vi "Run Test - Stop Condition (SubVI).vi"(8 "error in (no error)":errorcluster, 9 "Time":dbl, 11 "Cluster in":T2 {"M Event" items=["Stop", "Running", "PID", "Up Limit", "Down Limit", "Load Limit"]; "Test Type" items=["Please Select", "Triaxial Shear", "Triaxial UU", "Shearbox", "Permeability", "Consolidation (Stepped Loading)/Swelling", "Saturation (Incremental)", "User Defined", "UCT", "Isotropic Consolidation", "Swelling Pressure"]; "Data"."Test Type" items=["Please Select", "Triaxial Shear", "Triaxial UU", "Shearbox", "Permeability", "Consolidation (Stepped Loading)/Swelling", "Saturation (Incremental)", "User Defined", "UCT", "Isotropic Consolidation", "Swelling Pressure"]}) -> (0 "error out":errorcluster, 1 "Perm":T1, 2 "Delay":string, 3 "Cluster out":T2 {"M Event" items=["Stop", "Running", "PID", "Up Limit", "Down Limit", "Load Limit"]; "Test Type" items=["Please Select", "Triaxial Shear", "Triaxial UU", "Shearbox", "Permeability", "Consolidation (Stepped Loading)/Swelling", "Saturation (Incremental)", "User Defined", "UCT", "Isotropic Consolidation", "Swelling Pressure"]; "Data"."Test Type" items=["Please Select", "Triaxial Shear", "Triaxial UU", "Shearbox", "Permeability", "Consolidation (Stepped Loading)/Swelling", "Saturation (Incremental)", "User Defined", "UCT", "Isotropic Consolidation", "Swelling Pressure"]}, 5 "Enum":T11)   [LabVIEW 2019]
uses:
  Controls/RunTest - State.ctl
  Controls/RunTest - Data Structure.ctl
  Controls/Test Panel - Data Structure.ctl
  Controls/Station - Test Type.ctl
  <vilib>/Utility/miscctls.llb/LVRowAndColumnTypeDef.ctl
  Controls/RunTest - Calculate Data.ctl
  <vilib>/httpClient/ClientHandle.ctl
  Controls/RunTest - Start Condition.ctl
  Controls/RunTest - Stop Condition.ctl
  Controls/UDP - Event.ctl
  Controls/eFGV States.ctl
  <vilib>/httpClient/LabVIEWHTTPClient.lvlib
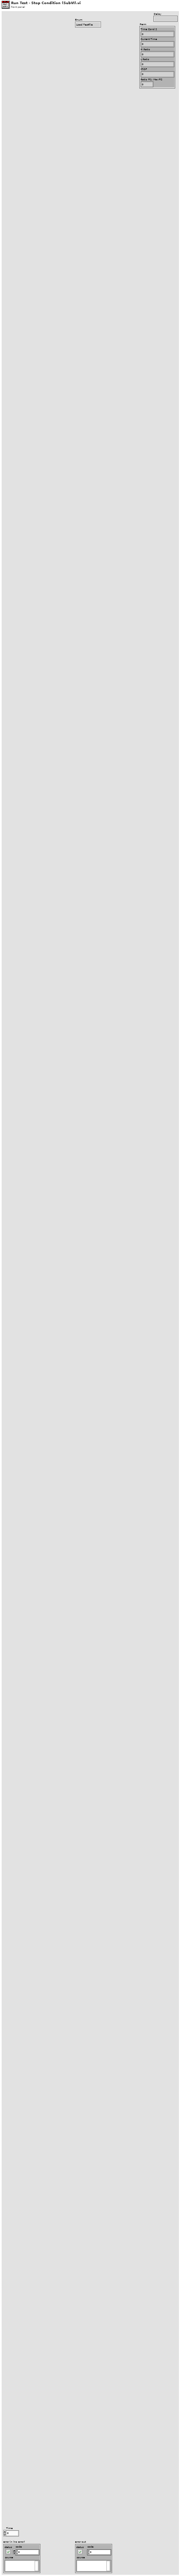
[diagram p1: front panel]
types:
  T1 = cluster{"Time Cond 2":dbl, "Current Time":dbl, "H Ratio":dbl, "L Ratio":dbl, "IF/OF":dbl, "Ratio =1; Max=2":u32}
  T2 = typedef "RunTest - Data Structure.ctl" = cluster{"Test Plan":string[], "PlanRow":i32, "Device Name":string[], "Timeout":i32, "Start?":bool, "Pause?":bool, "IP Address":string[], "LogRow":i32, "Logtype":u16, "Log Elapse":sgl, "Data":T3, "Stop log?":bool, "tdms":refnum<k34>, "Sensor Data":sgl[], "Start time":timestamp, "Prev Log Elapse":u32, "Plot":u16, "X-Axis":u16[], "Y-Axis":u16[], "XY":cluster{"X":dbl, "Y":dbl}[][], "End Stage?":bool, "1run":bool, "Condition":u16[], "Start Con":bool, "Log Con":bool, "Stop Con":bool, "Start Elapse":dbl, "Start Load":dbl, "Motor":i32, "StartRow":i32, "number log":i32, "Dir":bool, "Start time test":timestamp, "Auto":bool, "Check return?":bool, "Inv":cluster{"M":i32[], "Bool":bool[]}, "tdms temp":refnum<k34>, "Zero?":bool, "Plot Timer":dbl, "1st Run":bool, "TDMS Path":path, "MaxLoad":dbl, "Log Timer":sgl[], "Test Type":T4, "Log Sensor":string[], "Save?":bool, "1st Log":bool, "Y-Axis 2":u16[], "On Y-Axis 2":bool, "Decimal":u8[], "Init":cluster{"PWP TS":sgl, "Load TS":sgl, "Volume TS":sgl, "Disp TS":sgl, "CP":sgl, "Vol In":sgl, "Vol Out":sgl, "Load UCT":sgl, "Disp UCT":sgl, "PWP Sat":sgl, "CP Sat":sgl, "Volume IsoCons":sgl, "PWP IsoCons":sgl, "PWP TUU":sgl, "Load TUU":sgl, "Volume TUU":sgl, "Disp TUU":sgl, "Load Cons":sgl, "Disp Cons":sgl, "Volume Sat":sgl, "Vertical Load SB":sgl, "Vertical Disp SB":sgl, "H Disp SB":sgl, "H Load SB":sgl}, "Calc":T6, "Device Index":i32[], "Channel Index":i32[], "http ref":T7, "fileid":string, "Step Cons":cluster{"V Stress":sgl, "H Settlement":sgl}, "RunTest":bool, "Graph Last":i32, "Init?":bool, "Datalog":bool[], "Start":T8, "Stop":T9, "Running?":bool, "StartTime":dbl, "Log Prev Time":dbl, "KeyName":string[], "Test RunTime":dbl, "Log Prev Axial":dbl, "M Event":T10[], "Last Log":bool, "popup":bool, "PreStart UU":bool, "PreStart Sat":bool}
  T3 = typedef "Test Panel - Data Structure.ctl" = cluster{"Station":string, "Sample ID":string, "Job No":string, "Job Description":string, "Filename":string, "Test Type":T4, "Speciment No":string, "Depth":string, "Height":string, "Diameter/Length":string, "Weight":string, "Test Parameter":string, "Station[]":string[], "Edit Pos":T5, "Edit Pos Prev":T5, "Area":string, "Path":string}
  T4 = typedef "Station - Test Type.ctl" = u16
  T5 = typedef "LVRowAndColumnTypeDef.ctl" = cluster{"Row":i32, "Column":i32}
  T6 = typedef "RunTest - Calculate Data.ctl" = cluster{"TS":cluster{"Change PWP":sgl, "Change Vol":sgl, "Axial Load":sgl, "CiL":sgl, "Deviator":sgl, "Axial Strain":sgl, "MaxDeviator":sgl}, "TUU":cluster{"Change PWP":sgl, "Axial Load":sgl, "CiL":sgl, "Deviator":sgl, "Axial Strain":sgl, "MaxDeviator":sgl}, "Sat":cluster{"B Value":sgl, "PWP Diss":sgl, "CPP":sgl, "CV":sgl}, "Per":cluster{"Change Vol In":sgl, "Change Vol Out":sgl, "Mean Vol":sgl, "Gradient Pressure":sgl, "Outlet Flow":sgl, "Inlet Flow":sgl, "I X1":sgl, "I X2":sgl, "I Y1":sgl, "I Y2":sgl, "O X1":sgl, "O X2":sgl, "O Y1":sgl, "O Y2":sgl}, "Step Cons":cluster{"V Stress":sgl, "H Settlement":sgl, "Total H Settle":sgl, "Prev Total H":sgl}, "UCT":cluster{"ALC":sgl, "H Change":sgl, "Deviator":sgl, "Axial Strain":sgl, "V Stress":sgl, "MaxDeviator":sgl}, "ISO Cons":cluster{"CPP":sgl, "PWP Diss":sgl, "CV":sgl}, "SB":cluster{"Speci LenC":sgl, "Shear Strain":sgl, "H LC":sgl, "Normal Stress":sgl, "Shear Stress":sgl, "MaxShear":sgl}}
  T7 = typedef "LabVIEWHTTPClient.lvlib/ClientHandle.ctl" = refnum<k1>
  T8 = typedef "RunTest - Start Condition.ctl" = cluster{"Cons":cluster{"VS":dbl, "Delay":bool, "No Delay":dbl}, "Sat":cluster{"CP":dbl, "BP":dbl, "StartBP":bool, "Target CP":bool, "Target BP":bool}, "Iso":cluster{"Select":dbl, "BP":dbl, "IC2":dbl, "IC3":dbl, "IC4":dbl, ". IC6":bool, "IC6":dbl, "IC6-2":dbl, "Target":bool, "Time Cond":dbl, "Last PWP":dbl}, "TS":cluster{"SS":dbl, "Engage":bool, "ES":dbl, "LC":dbl, "PreStart":bool, "Trig SS":bool, "Drain":dbl}, "TUU":cluster{"SS":dbl, "Engage":bool, "ES":dbl, "LC":dbl, "PreStart":bool, "Trig SS":bool, "CP":dbl, "Delay Value":dbl, "Delay":bool, "CP PID":bool}, "UCT":cluster{"SS":dbl, "Engage":bool, "ES":dbl, "LC":dbl, "PreStart":bool, "Trig SS":bool}, "Enable?":bool, "SB":cluster{"SS":dbl, "Engage":bool, "ES":dbl, "LC":dbl, "PreStart":bool, "Trig SS":bool, "VS":dbl, "Delay Value":dbl, "Delay":bool, "VS PID":bool}, "Perm":cluster{"DP":dbl}}
  T9 = typedef "RunTest - Stop Condition.ctl" = cluster{"Cons":cluster{"Select":i32, "Disp":dbl, "Time":dbl, "Time2":dbl, "Disp 2":dbl, "Time Cond":dbl, "Last Disp":dbl, "Swell":bool}, "Sat":cluster{"Select":i32, "PP":dbl, "Time":dbl, "VC":dbl, "Time2":dbl, "Time Cond":dbl, "Last PP":dbl, ".B":bool, "B":dbl, "Last Vc":dbl, "Time Cond 2":dbl, "Time3":dbl, "Time Cond 3":dbl, "B Achieve":bool}, "Iso":cluster{"PP":dbl, "Time":dbl, "VC":dbl, "Time2":dbl, "Time Cond":dbl, "Last Vc":dbl, ".PP":bool, "Time Cond 2":dbl, "Select":i32}, "TS":cluster{"Axial":dbl, ".MaxDev":bool, "MaxDev Value":dbl, "Return":bool, "Reset":bool, "Prev Time":dbl, "PostStop Run":bool, "CP Stop":bool, "BP Stop":bool, "PostStop Trig":bool, "Reset Value":dbl, "BPTrig":bool, "CPTrig":bool, "VLCTrig":bool}, "TUU":cluster{"Axial":dbl, ".MaxDev":bool, "MaxDev Value":dbl, "Return":bool, "Reset":bool, "Prev Time":dbl, "PostStop Run":bool, "CP Stop":bool, "BP Stop":bool, "PostStop Trig":bool, "Reset Value":dbl, "BPTrig":bool, "CPTrig":bool, "VLCTrig":bool}, "UCT":cluster{"Axial":dbl, ".MaxDev":bool, "MaxDev Value":dbl, "Return":bool, "Reset":bool, "Prev Time":dbl, "PostStop Run":bool, "CP Stop":bool, "BP Stop":bool, "PostStop Trig":bool}, "Enable?":bool, "SB":cluster{"Shear":dbl, ".MaxShear":bool, "MaxShear Value":dbl, "Return":bool, "Reset":bool, "Prev Time":dbl, "PostStop Run":bool, "CP Stop":bool, "BP Stop":bool, "PostStop Trig":bool, "Reset Value":dbl, "BPTrig":bool, "CPTrig":bool, "VLCTrig":bool}, "Perm":cluster{"Max Time":bool, "Reset":bool, "PostStop Run":bool, "Ratio":bool, "Reset Value":dbl, "Time":dbl, "RatioTime":dbl, "RatioMore":dbl, "RatioLess":dbl, "Time Cond":dbl, "Time Cond 2":dbl, "Prev IF":dbl, "Prev OF":dbl, "PostStop Trig":bool, "BP Trig":bool, "DP Stop":bool, "BP Stop":bool, "CP Stop":bool, "CP Trig":bool}, "SP":cluster{".Max Time":bool, ".Time":bool, "Time":dbl, "MaxTime":dbl, "Time Cond":dbl, "Max Time Cond":dbl, "Stress":dbl}}
  T10 = typedef "UDP - Event.ctl" = u16
  T11 = typedef "RunTest - State.ctl" = enum16{"Load Testfile", "Notifier", "Init", "Idle", "Load", "Read DB", "Run", "Pause", "Stop", "Check Start", "Check Stop", "Check Post Stop", "Check Log", "EndStage", "Data View", "Display", "Graph", "Graph Old", "Close", "Stop PID", "Check Limit", "Auto", "Up", "Log", "Zero", "Machine Control", "Save Report"}
  T12 = typedef "eFGV States.ctl" = enum16{"Init", "Read", "Write", "Exit"}
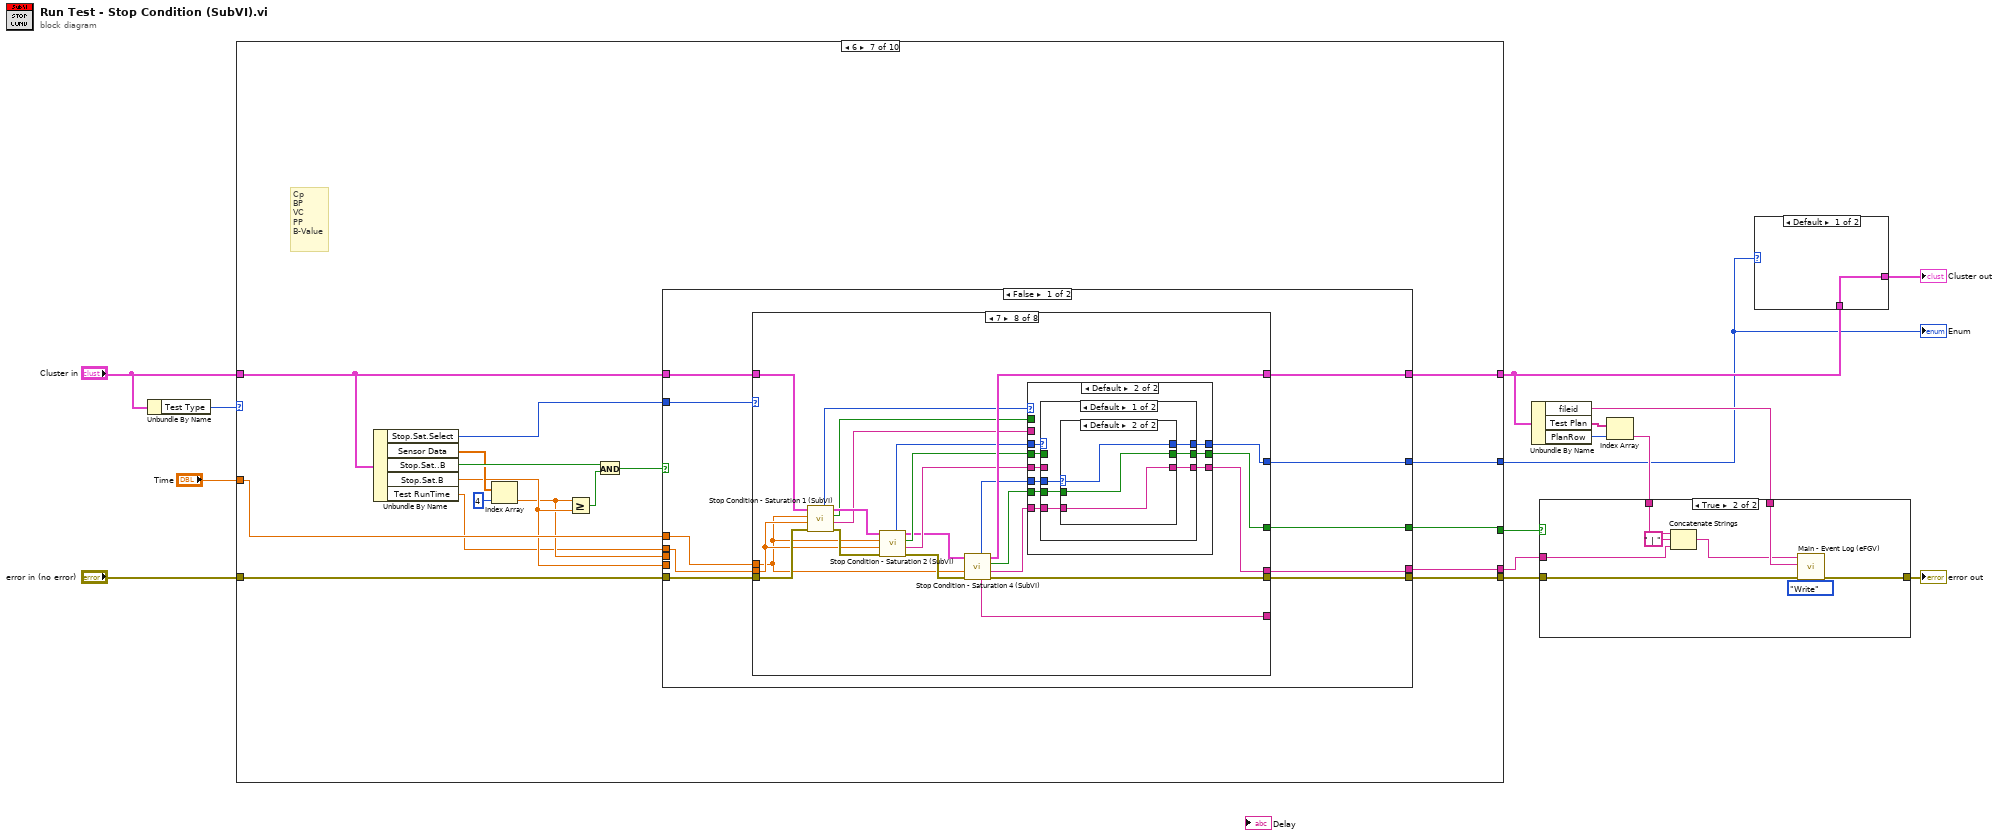
[diagram p0: block diagram]
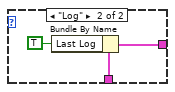
[diagram p2: hidden frame]
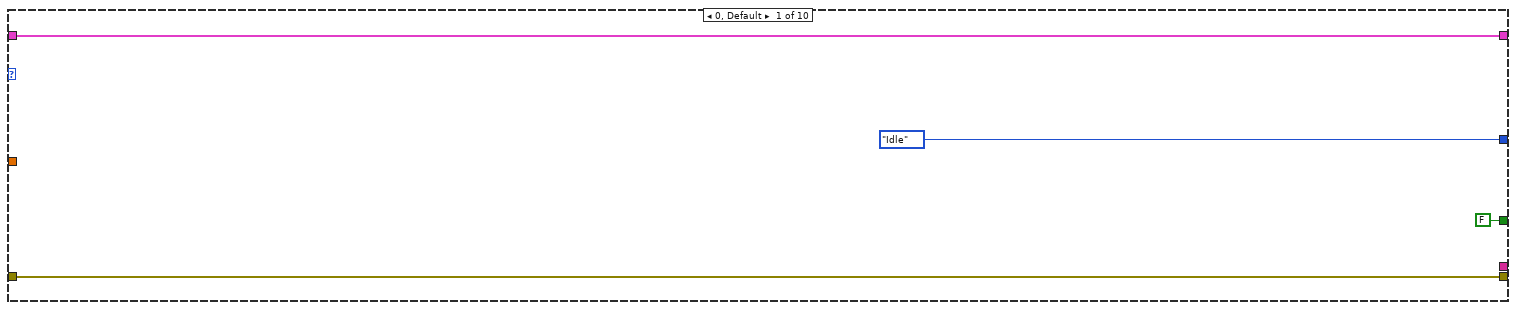
[diagram p3: hidden frame]
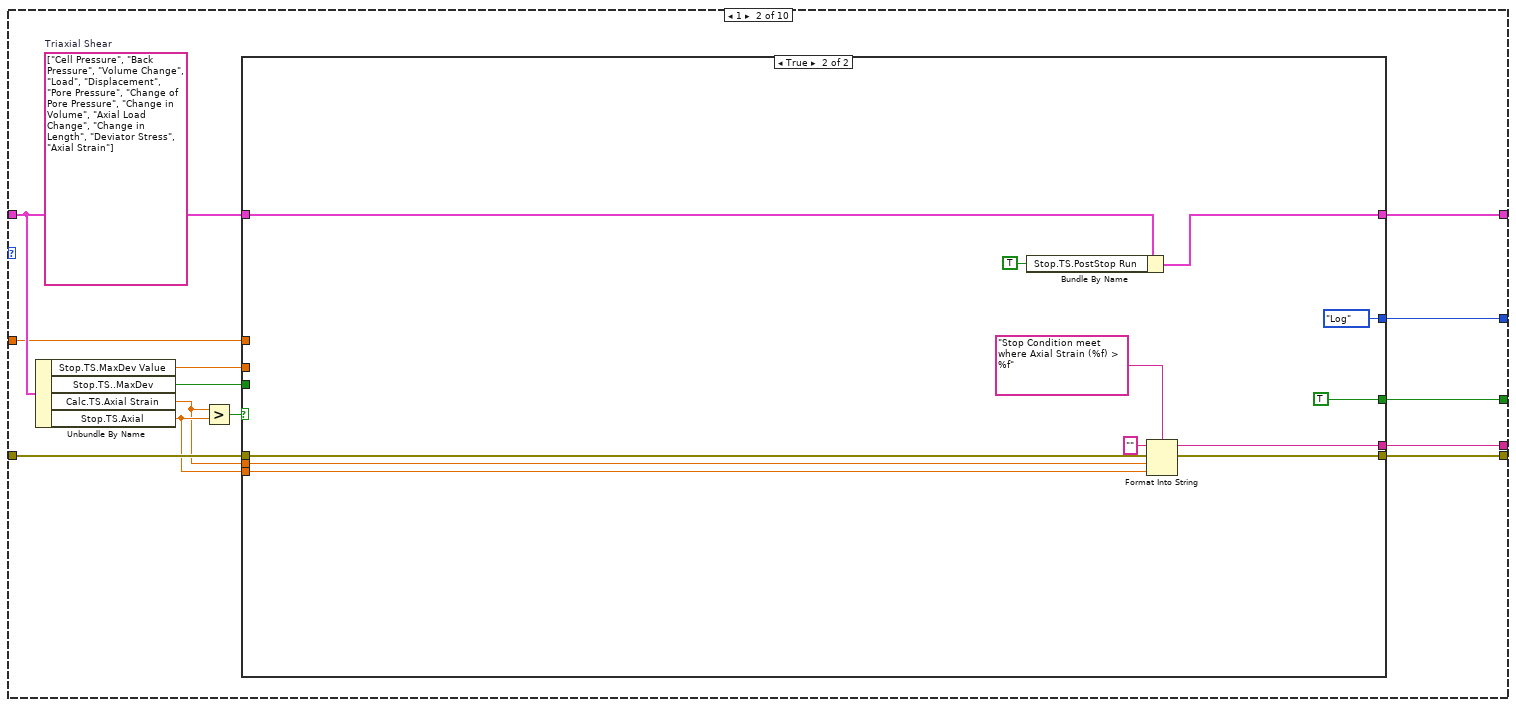
[diagram p4: hidden frame]
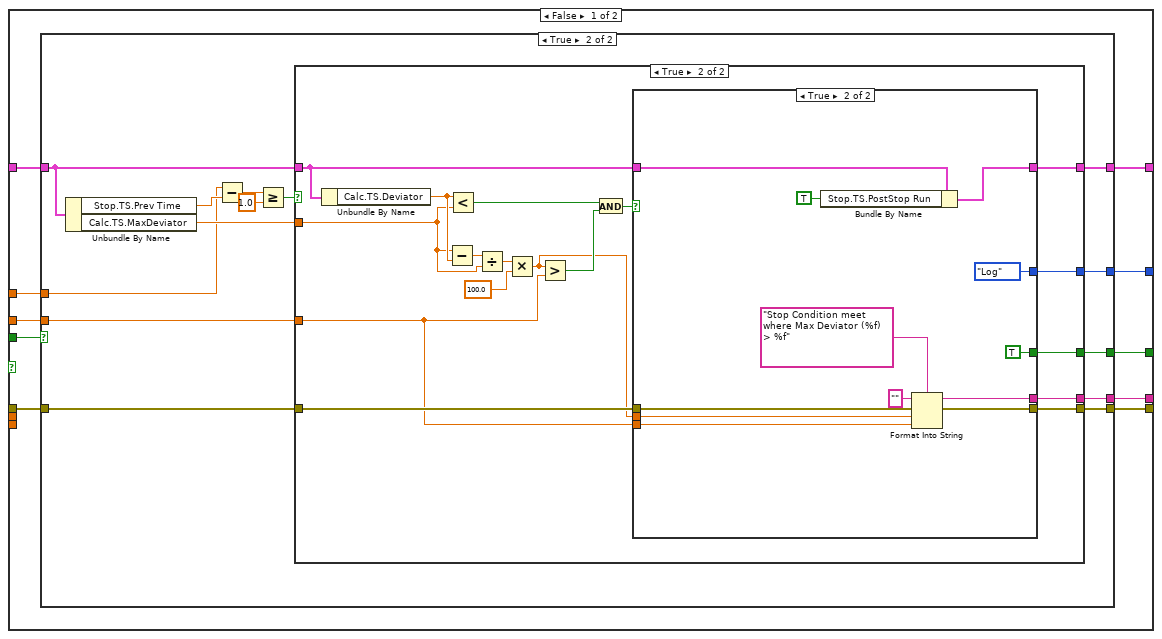
[diagram p5: hidden frame]
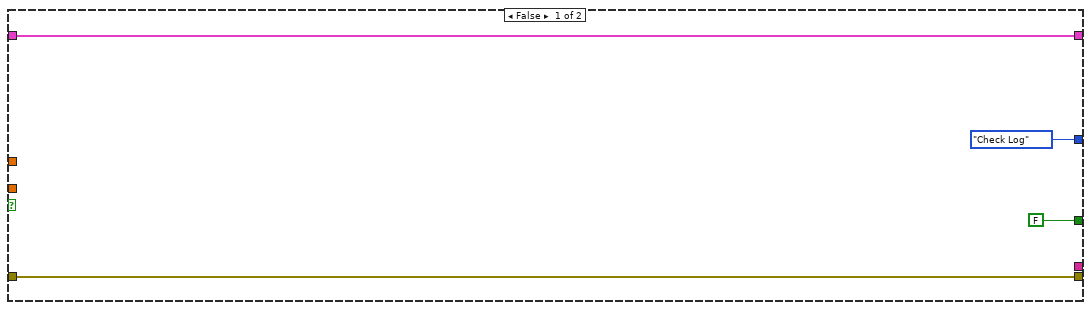
[diagram p6: hidden frame]
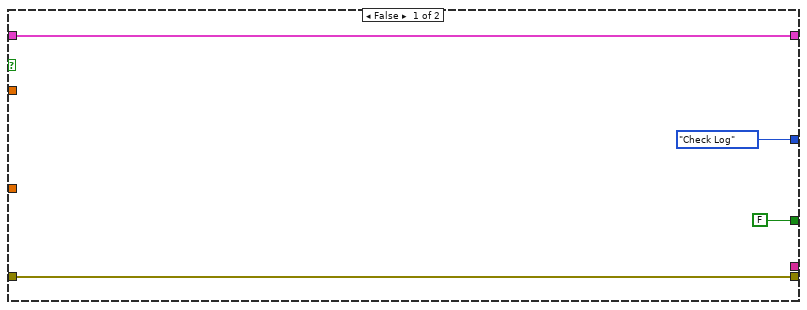
[diagram p7: hidden frame]
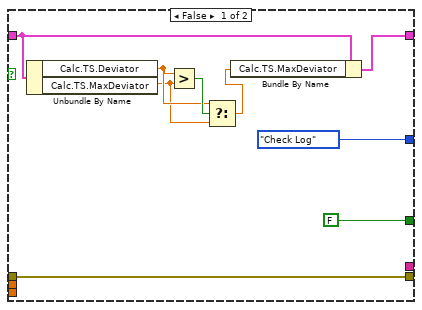
[diagram p8: hidden frame]
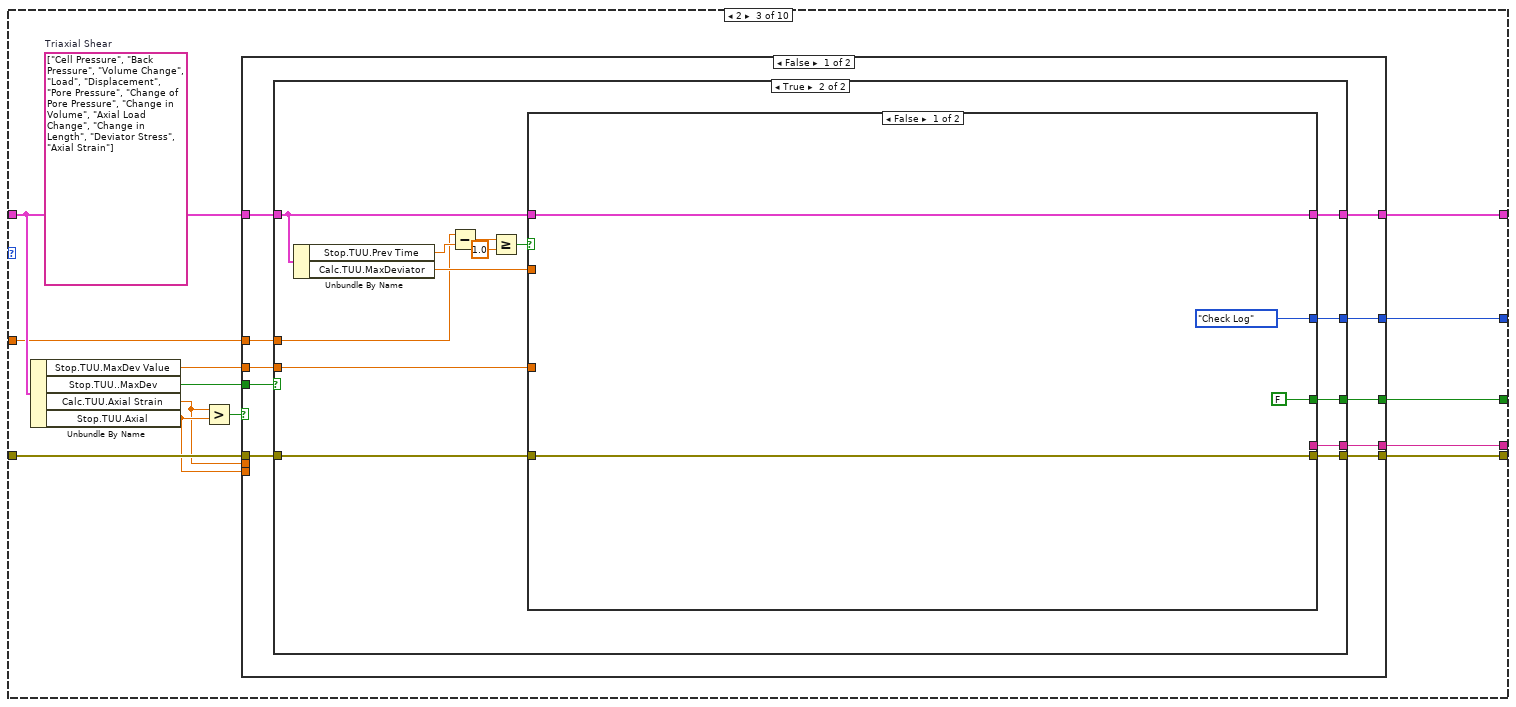
[diagram p9: hidden frame]
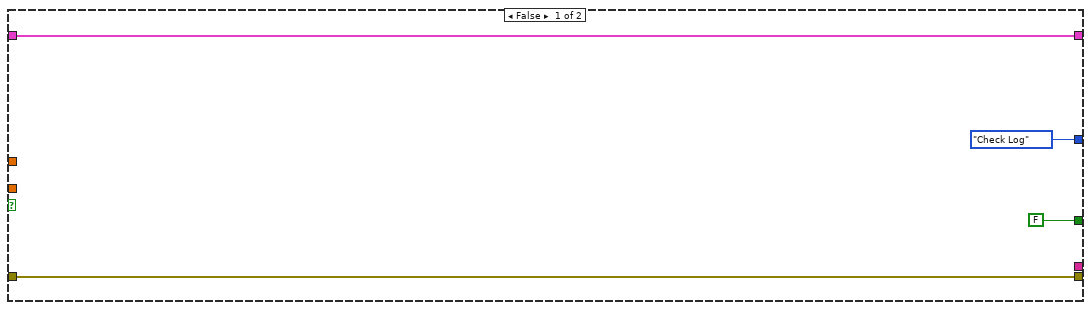
[diagram p10: hidden frame]
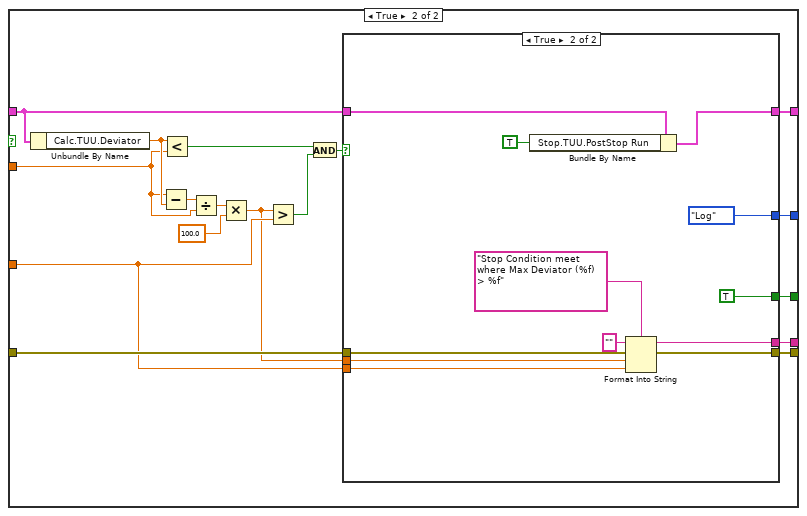
[diagram p11: hidden frame]
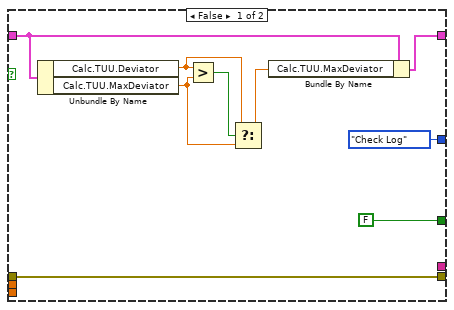
[diagram p12: hidden frame]
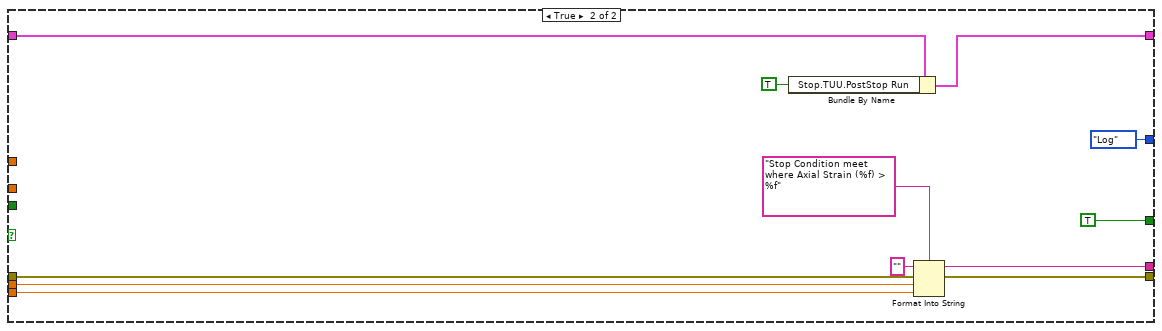
[diagram p13: hidden frame]
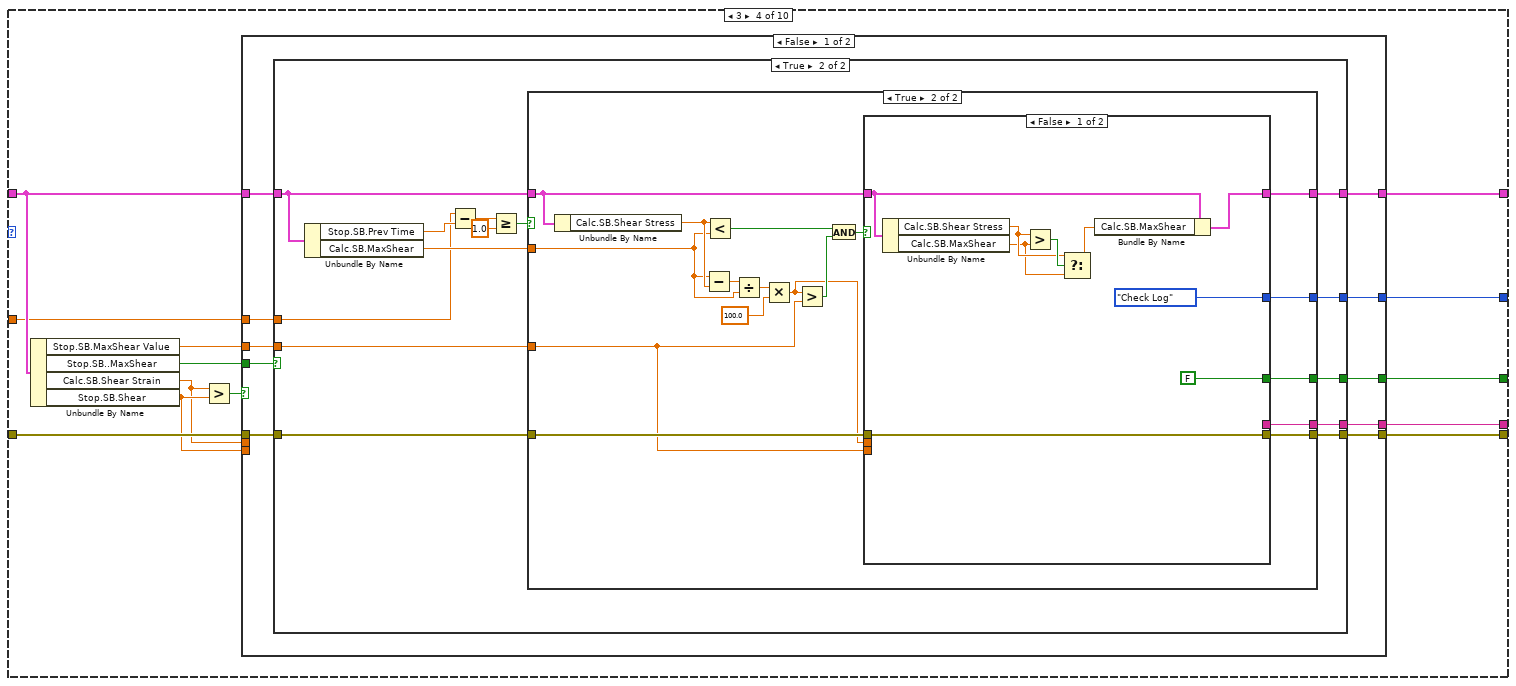
[diagram p14: hidden frame]
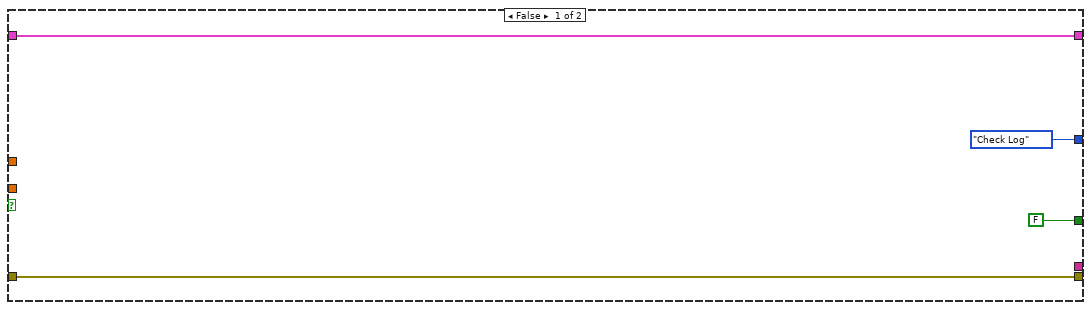
[diagram p15: hidden frame]
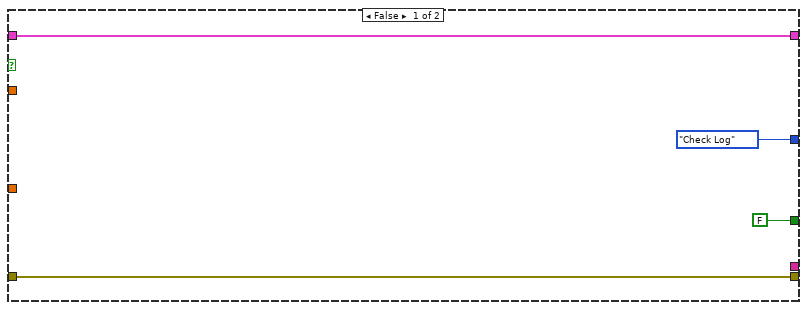
[diagram p16: hidden frame]
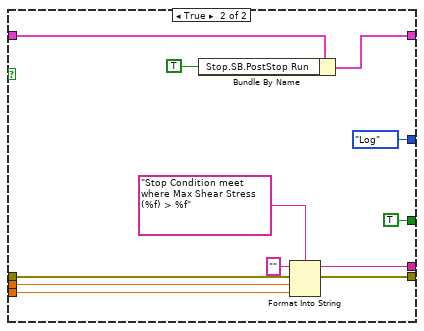
[diagram p17: hidden frame]
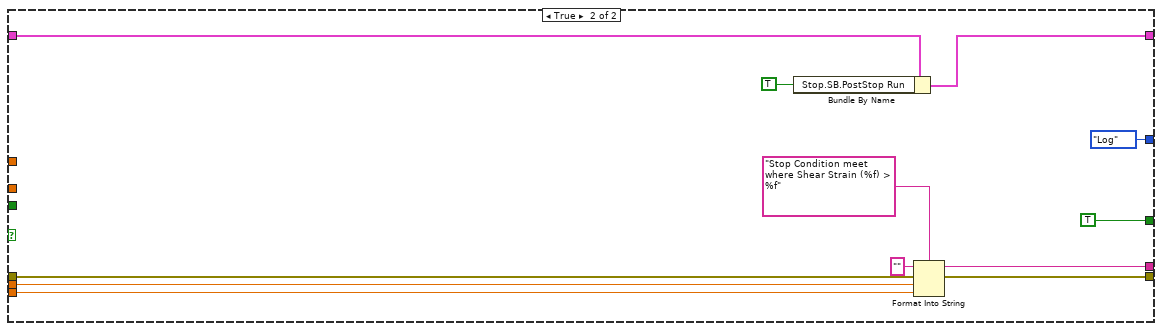
[diagram p18: hidden frame]
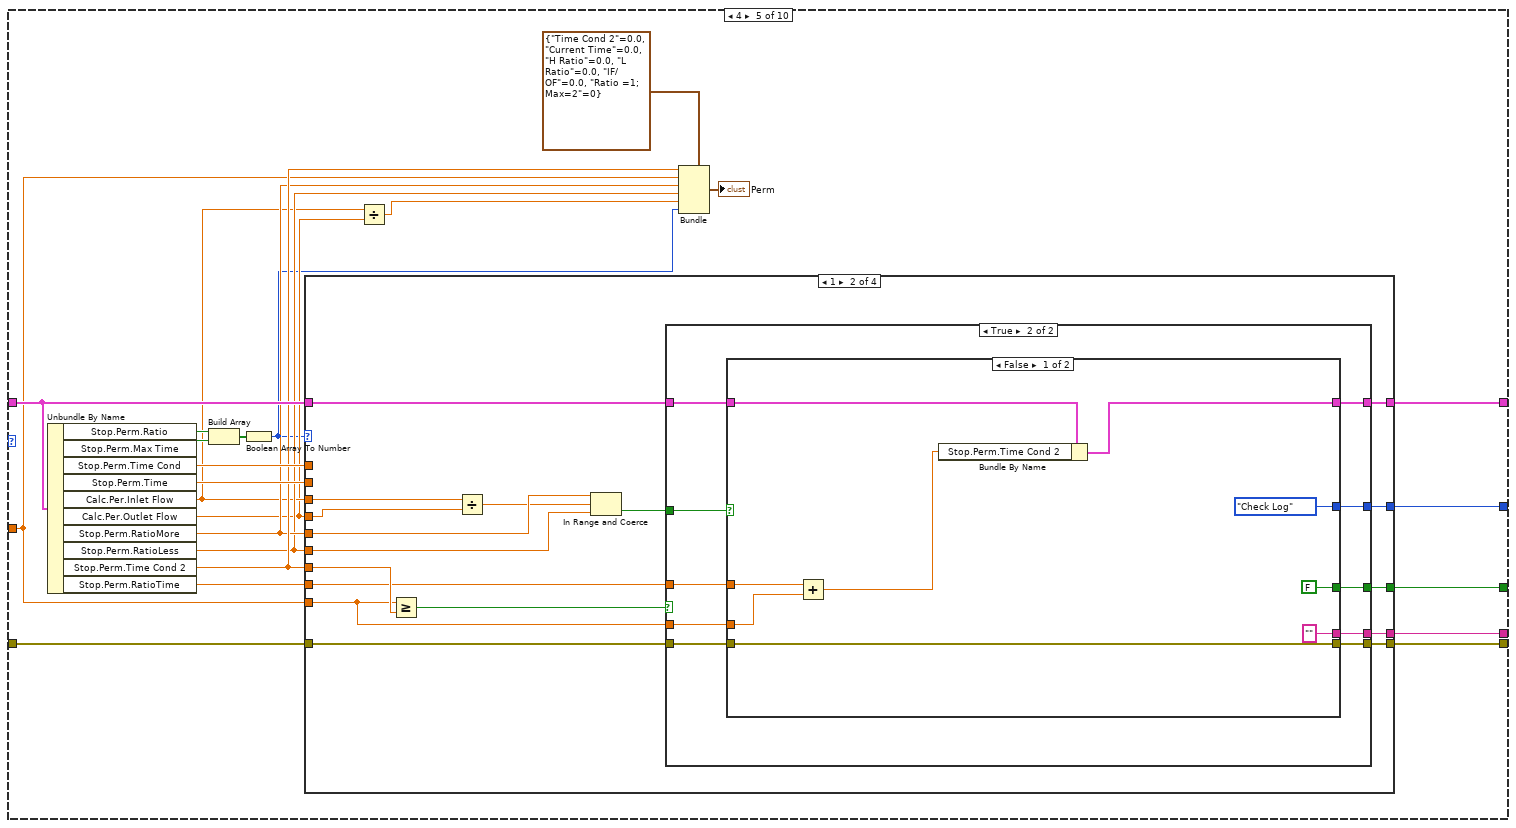
[diagram p19: hidden frame]
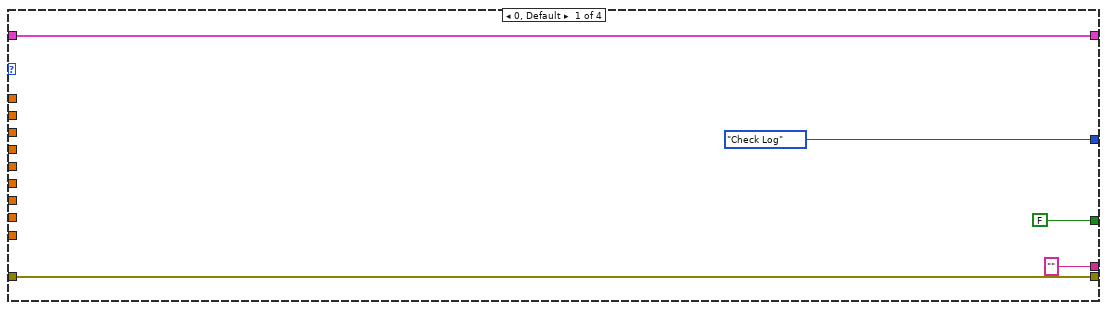
[diagram p20: hidden frame]
diagram:
  n1 = Unbundle By Name("Cluster in") -> ("Test Type"=w4:T4)
  n2 = case shown="6" w4 {
    tunnel: [w19 w31 w127 w222 w324 w524 w859 w1083 w1177 w1422] -> w2
    tunnel: "Cluster in" -> [w19 w30 w126 w221 w323 w523 w858 w1082 w1176 w1421]
    tunnel: [w18 w29 w125 w220 w327 w527 w862 w1081 w1180 w1425] -> w7
    tunnel: "error in (no error)" -> [w18 w28 w124 w219 w326 w526 w861 w1080 w1179 w1424]
    tunnel: [RunTest_-_State."Idle" w22 w118 w213 w325 w525 w860 w1074 w1178 w1423] -> w1
    tunnel: [_ w27 w123 w218 w322 w522 w857 w1079 w1169 w1420] -> w10
    tunnel: [FALSE w26 w122 w217 w321 w516 w856 w1078 w1168 w1419] -> w11
    tunnel: "Time" -> [_ w20 w116 w211 w312 w514 w855 w1072 w1167 w1418]
    frame 0, Default {
    }
    frame 1 {
      (unwired) string[] ["Cell Pressure", "Back Pressure", "Volume Change", "Load", "Displacement", "Pore Pressure", "Change of Pore Pressure", "Change in Volume", "Axial Load Change", "Change in Length", "Deviator Stress", "Axial Strain"]  # Triaxial Shear
      n3 = Unbundle By Name(w30) -> ("Stop.TS.MaxDev Value"=w21:dbl, "Stop.TS..MaxDev"=w23:bool, "Calc.TS.Axial Strain"=w24:sgl, "Stop.TS.Axial"=w25:dbl)
      n4 = Greater?(x=w24, y=w25) -> (0:w32:bool)
      n5 = case shown="True" w32 {
        tunnel: [w39 w104] -> w31
        tunnel: w30 -> [w38 w103]
        tunnel: [w41 w113] -> w29
        tunnel: w28 -> [w40 w112]
        tunnel: [w34 w110] -> w27
        tunnel: [w36 TRUE] -> w26
        tunnel: w25 -> [_ w108]
        tunnel: w24 -> [_ w107]
        tunnel: w23 -> [w42 _]
        tunnel: [w37 RunTest_-_State."Log"] -> w22
        tunnel: w21 -> [w35 _]
        tunnel: w20 -> [w33 _]
        frame False {
          n6 = case shown="True" w42 {
            tunnel: [w46 w54] -> w41
            tunnel: w40 -> [w46 w53]
            tunnel: [w43 w56] -> w39
            tunnel: w38 -> [w43 w55]
            tunnel: [RunTest_-_State."Check Log" w52] -> w37
            tunnel: [FALSE w51] -> w36
            tunnel: w35 -> [_ w49]
            tunnel: [_ w48] -> w34
            tunnel: w33 -> [_ w47]
            frame False {
            }
            frame True {
              n7 = Unbundle By Name(w55) -> ("Stop.TS.Prev Time"=w60:dbl, "Calc.TS.MaxDeviator"=w50:sgl)
              n8 = Subtract(x=w47, y=w60) -> (x-y=w59:dbl)
              n9 = Greater Or Equal?(x=w59, y=1.0) -> (x >= y?=w57:bool)
              n10 = case shown="True" w57 {
                tunnel: [w63 w81] -> w56
                tunnel: w55 -> [w63 w80]
                tunnel: [w62 w77] -> w54
                tunnel: w53 -> [w62 w76]
                tunnel: [RunTest_-_State."Check Log" w79] -> w52
                tunnel: [FALSE w78] -> w51
                tunnel: w50 -> [_ w68]
                tunnel: w49 -> [_ w67]
                tunnel: [_ w66] -> w48
                frame False {
                }
                frame True {
                  n11 = Unbundle By Name(w80) -> ("Calc.TS.Deviator"=w75:sgl)
                  n12 = Subtract(x=w68, y=w75) -> (x-y=w74:sgl)
                  n13 = Less?(x=w75, y=w68) -> (x < y?=w71:bool)
                  n14 = Divide(x=w74, y=w68) -> (x/y=w73:sgl)
                  n15 = Multiply(x=w73, y=sgl 100.0) -> (x*y=w65:sgl)
                  n16 = Greater?(x=w65, y=w67) -> (0:w70:bool)
                  n17 = And(x=w71, y=w70) -> (x .and. y?=w69:bool)
                  n18 = case shown="True" w69 {
                    tunnel: [w87 w92] -> w81
                    tunnel: w80 -> [w86 w91]
                    tunnel: [RunTest_-_State."Check Log" RunTest_-_State."Log"] -> w79
                    tunnel: [FALSE TRUE] -> w78
                    tunnel: [w88 w97] -> w77
                    tunnel: w76 -> [w88 w98]
                    tunnel: w65 -> [_ w96]
                    tunnel: w67 -> [_ w95]
                    tunnel: [_ w94] -> w66
                    frame False {
                      n19 = Unbundle By Name(w86) -> ("Calc.TS.Deviator"=w84:sgl, "Calc.TS.MaxDeviator"=w83:sgl)
                      n20 = Greater?(x=w84, y=w83) -> (0:w85:bool)
                      n21 = Select(t=w84, s=w85, f=w83) -> (s? t:f=w82:sgl)
                      n22 = Bundle By Name(cluster=w86, "Calc.TS.MaxDeviator"=w82) -> (w87:T2)
                    }
                    frame True {
                      n23 = Bundle By Name(cluster=w91, "Stop.TS.PostStop Run"=TRUE) -> (w92:T2)
                      n24 = Format Into String(format string="Stop Condition meet where Max Deviator (%f) > %f", initial string="", error in=w98, w96, w95) -> (resulting string=w94:string, error out=w97:errorcluster)
                    }
                  }
                }
              }
            }
          }
        }
        frame True {
          n25 = Bundle By Name(cluster=w103, "Stop.TS.PostStop Run"=TRUE) -> (w104:T2)
          n26 = Format Into String(format string="Stop Condition meet where Axial Strain (%f) > %f", initial string="", error in=w112, w107, w108) -> (resulting string=w110:string, error out=w113:errorcluster)
        }
      }
    }
    frame 2 {
      (unwired) string[] ["Cell Pressure", "Back Pressure", "Volume Change", "Load", "Displacement", "Pore Pressure", "Change of Pore Pressure", "Change in Volume", "Axial Load Change", "Change in Length", "Deviator Stress", "Axial Strain"]  # Triaxial Shear
      n27 = Unbundle By Name(w126) -> ("Stop.TUU.MaxDev Value"=w117:dbl, "Stop.TUU..MaxDev"=w119:bool, "Calc.TUU.Axial Strain"=w120:sgl, "Stop.TUU.Axial"=w121:dbl)
      n28 = Greater?(x=w120, y=w121) -> (0:w115:bool)
      n29 = case shown="False" w115 {
        tunnel: [w134 w199] -> w127
        tunnel: w126 -> [w133 w198]
        tunnel: [w136 w208] -> w125
        tunnel: w124 -> [w135 w207]
        tunnel: [w129 w205] -> w123
        tunnel: [w131 TRUE] -> w122
        tunnel: w121 -> [_ w203]
        tunnel: w120 -> [_ w202]
        tunnel: w119 -> [w137 _]
        tunnel: [w132 RunTest_-_State."Log"] -> w118
        tunnel: w117 -> [w130 _]
        tunnel: w116 -> [w128 _]
        frame False {
          n30 = case shown="True" w137 {
            tunnel: [w141 w149] -> w136
            tunnel: w135 -> [w141 w148]
            tunnel: [w138 w151] -> w134
            tunnel: w133 -> [w138 w150]
            tunnel: [RunTest_-_State."Check Log" w147] -> w132
            tunnel: [FALSE w146] -> w131
            tunnel: w130 -> [_ w144]
            tunnel: [_ w143] -> w129
            tunnel: w128 -> [_ w142]
            frame False {
            }
            frame True {
              n31 = Unbundle By Name(w150) -> ("Stop.TUU.Prev Time"=w155:dbl, "Calc.TUU.MaxDeviator"=w145:sgl)
              n32 = Subtract(x=w142, y=w155) -> (x-y=w154:dbl)
              n33 = Greater Or Equal?(x=w154, y=1.0) -> (x >= y?=w152:bool)
              n34 = case shown="False" w152 {
                tunnel: [w158 w176] -> w151
                tunnel: w150 -> [w158 w175]
                tunnel: [w157 w172] -> w149
                tunnel: w148 -> [w157 w171]
                tunnel: [RunTest_-_State."Check Log" w174] -> w147
                tunnel: [FALSE w173] -> w146
                tunnel: w145 -> [_ w163]
                tunnel: w144 -> [_ w162]
                tunnel: [_ w161] -> w143
                frame False {
                }
                frame True {
                  n35 = Unbundle By Name(w175) -> ("Calc.TUU.Deviator"=w170:sgl)
                  n36 = Subtract(x=w163, y=w170) -> (x-y=w169:sgl)
                  n37 = Less?(x=w170, y=w163) -> (x < y?=w166:bool)
                  n38 = Divide(x=w169, y=w163) -> (x/y=w168:sgl)
                  n39 = Multiply(x=w168, y=sgl 100.0) -> (x*y=w160:sgl)
                  n40 = Greater?(x=w160, y=w162) -> (0:w165:bool)
                  n41 = And(x=w166, y=w165) -> (x .and. y?=w164:bool)
                  n42 = case shown="True" w164 {
                    tunnel: [w182 w187] -> w176
                    tunnel: w175 -> [w181 w186]
                    tunnel: [RunTest_-_State."Check Log" RunTest_-_State."Log"] -> w174
                    tunnel: [FALSE TRUE] -> w173
                    tunnel: [w183 w192] -> w172
                    tunnel: w171 -> [w183 w193]
                    tunnel: w160 -> [_ w191]
                    tunnel: w162 -> [_ w190]
                    tunnel: [_ w189] -> w161
                    frame False {
                      n43 = Unbundle By Name(w181) -> ("Calc.TUU.Deviator"=w179:sgl, "Calc.TUU.MaxDeviator"=w178:sgl)
                      n44 = Greater?(x=w179, y=w178) -> (0:w180:bool)
                      n45 = Select(t=w179, s=w180, f=w178) -> (s? t:f=w177:sgl)
                      n46 = Bundle By Name(cluster=w181, "Calc.TUU.MaxDeviator"=w177) -> (w182:T2)
                    }
                    frame True {
                      n47 = Bundle By Name(cluster=w186, "Stop.TUU.PostStop Run"=TRUE ("Stop.TS.PostStop Run")) -> (w187:T2)
                      n48 = Format Into String(format string="Stop Condition meet where Max Deviator (%f) > %f", initial string="", error in=w193, w191, w190) -> (resulting string=w189:string, error out=w192:errorcluster)
                    }
                  }
                }
              }
            }
          }
        }
        frame True {
          n49 = Bundle By Name(cluster=w198, "Stop.TUU.PostStop Run"=TRUE ("Stop.TS.PostStop Run")) -> (w199:T2)
          n50 = Format Into String(format string="Stop Condition meet where Axial Strain (%f) > %f", initial string="", error in=w207, w202, w203) -> (resulting string=w205:string, error out=w208:errorcluster)
        }
      }
    }
    frame 3 {
      n51 = Unbundle By Name(w221) -> ("Stop.SB.MaxShear Value"=w212:dbl, "Stop.SB..MaxShear"=w214:bool, "Calc.SB.Shear Strain"=w215:sgl, "Stop.SB.Shear"=w216:dbl)
      n52 = Greater?(x=w215, y=w216) -> (0:w210:bool)
      n53 = case shown="False" w210 {
        tunnel: [w229 w294] -> w222
        tunnel: w221 -> [w228 w293]
        tunnel: [w231 w303] -> w220
        tunnel: w219 -> [w230 w302]
        tunnel: [w224 w300] -> w218
        tunnel: [w226 TRUE] -> w217
        tunnel: w216 -> [_ w298]
        tunnel: w215 -> [_ w297]
        tunnel: w214 -> [w232 _]
        tunnel: [w227 RunTest_-_State."Log"] -> w213
        tunnel: w212 -> [w225 _]
        tunnel: w211 -> [w223 _]
        frame False {
          n54 = case shown="True" w232 {
            tunnel: [w236 w244] -> w231
            tunnel: w230 -> [w236 w243]
            tunnel: [w233 w246] -> w229
            tunnel: w228 -> [w233 w245]
            tunnel: [RunTest_-_State."Check Log" w242] -> w227
            tunnel: [FALSE w241] -> w226
            tunnel: w225 -> [_ w239]
            tunnel: [_ w238] -> w224
            tunnel: w223 -> [_ w237]
            frame False {
            }
            frame True {
              n55 = Unbundle By Name(w245) -> ("Stop.SB.Prev Time"=w250:dbl, "Calc.SB.MaxShear"=w240:sgl)
              n56 = Subtract(x=w237, y=w250) -> (x-y=w249:dbl)
              n57 = Greater Or Equal?(x=w249, y=1.0) -> (x >= y?=w247:bool)
              n58 = case shown="True" w247 {
                tunnel: [w253 w271] -> w246
                tunnel: w245 -> [w253 w270]
                tunnel: [w252 w267] -> w244
                tunnel: w243 -> [w252 w266]
                tunnel: [RunTest_-_State."Check Log" w269] -> w242
                tunnel: [FALSE w268] -> w241
                tunnel: w240 -> [_ w258]
                tunnel: w239 -> [_ w257]
                tunnel: [_ w256] -> w238
                frame False {
                }
                frame True {
                  n59 = Unbundle By Name(w270) -> ("Calc.SB.Shear Stress"=w265:sgl)
                  n60 = Subtract(x=w258, y=w265) -> (x-y=w264:sgl)
                  n61 = Less?(x=w265, y=w258) -> (x < y?=w261:bool)
                  n62 = Divide(x=w264, y=w258) -> (x/y=w263:sgl)
                  n63 = Multiply(x=w263, y=sgl 100.0) -> (x*y=w255:sgl)
                  n64 = Greater?(x=w255, y=w257) -> (0:w260:bool)
                  n65 = And(x=w261, y=w260) -> (x .and. y?=w259:bool)
                  n66 = case shown="False" w259 {
                    tunnel: [w277 w282] -> w271
                    tunnel: w270 -> [w276 w281]
                    tunnel: [RunTest_-_State."Check Log" RunTest_-_State."Log"] -> w269
                    tunnel: [FALSE TRUE] -> w268
                    tunnel: [w278 w287] -> w267
                    tunnel: w266 -> [w278 w288]
                    tunnel: w255 -> [_ w286]
                    tunnel: w257 -> [_ w285]
                    tunnel: [_ w284] -> w256
                    frame False {
                      n67 = Unbundle By Name(w276) -> ("Calc.SB.Shear Stress"=w274:sgl, "Calc.SB.MaxShear"=w273:sgl)
                      n68 = Greater?(x=w274, y=w273) -> (0:w275:bool)
                      n69 = Select(t=w274, s=w275, f=w273) -> (s? t:f=w272:sgl)
                      n70 = Bundle By Name(cluster=w276, "Calc.SB.MaxShear"=w272) -> (w277:T2)
                    }
                    frame True {
                      n71 = Bundle By Name(cluster=w281, "Stop.SB.PostStop Run"=TRUE ("Stop.TS.PostStop Run")) -> (w282:T2)
                      n72 = Format Into String(format string="Stop Condition meet where Max Shear Stress (%f) > %f", initial string="", error in=w288, w286, w285) -> (resulting string=w284:string, error out=w287:errorcluster)
                    }
                  }
                }
              }
            }
          }
        }
        frame True {
          n73 = Bundle By Name(cluster=w293, "Stop.SB.PostStop Run"=TRUE ("Stop.TS.PostStop Run")) -> (w294:T2)
          n74 = Format Into String(format string="Stop Condition meet where Shear Strain (%f) > %f", initial string="", error in=w302, w297, w298) -> (resulting string=w300:string, error out=w303:errorcluster)
        }
      }
    }
    frame 4 {
      n75 = Unbundle By Name(w323) -> ("Stop.Perm.Ratio"=w320:bool, "Stop.Perm.Max Time"=w319:bool, "Stop.Perm.Time Cond"=w317:dbl, "Stop.Perm.Time"=w316:dbl, "Calc.Per.Inlet Flow"=w309:sgl, "Calc.Per.Outlet Flow"=w308:sgl, "Stop.Perm.RatioMore"=w311:dbl, "Stop.Perm.RatioLess"=w310:dbl, "Stop.Perm.Time Cond 2"=w313:dbl, "Stop.Perm.RatioTime"=w315:dbl)
      n76 = Build Array(w320, w319) -> (w318:bool[])
      n77 = Boolean Array To Number(Boolean array=w318) -> (number=w306:u32)
      n78 = case shown="1" w306 {
        tunnel: [w328 w337 w389 w421] -> w327
        tunnel: w326 -> [w328 w336 w390 w420]
        tunnel: [RunTest_-_State."Check Log" w349 w396 w433] -> w325
        tunnel: [w329 w339 w386 w423] -> w324
        tunnel: w323 -> [w329 w338 w387 w422]
        tunnel: ["" w348 w395 w432] -> w322
        tunnel: [FALSE w347 w394 w431] -> w321
        tunnel: w312 -> [_ w334 w393 w418]
        tunnel: w317 -> [_ _ w392 w417]
        tunnel: w316 -> [_ _ w388 w415]
        tunnel: w309 -> [_ w346 _ w430]
        tunnel: w308 -> [_ w345 _ w429]
        tunnel: w311 -> [_ w344 _ w428]
        tunnel: w310 -> [_ w343 _ w427]
        tunnel: w313 -> [_ w341 _ w425]
        tunnel: w315 -> [_ w335 _ w419]
        frame 0, Default {
        }
        frame 1 {
          n79 = Greater Or Equal?(x=w334, y=w341) -> (x >= y?=w333:bool)
          n80 = Divide(x=w346, y=w345) -> (x/y=w342:sgl)
          n81 = In Range and Coerce(upper limit=w344, x=w342, lower limit=w343) -> (In Range?=w340:bool)  [unwired: 1 out]
          n82 = case shown="True" w333 {
            tunnel: [RunTest_-_State."Check Log" w364] -> w349
            tunnel: ["" w363] -> w348
            tunnel: [FALSE w362] -> w347
            tunnel: w340 -> [_ w361]
            tunnel: [w354 w360] -> w339
            tunnel: w338 -> [w354 w359]
            tunnel: [w351 w358] -> w337
            tunnel: w336 -> [w351 w357]
            tunnel: w335 -> [_ w356]
            tunnel: w334 -> [_ w355]
            frame False {
            }
            frame True {
              n83 = case shown="False" w361 {
                tunnel: [RunTest_-_State."Check Log" RunTest_-_State."Log"] -> w364
                tunnel: ["" w384] -> w363
                tunnel: [FALSE TRUE] -> w362
                tunnel: [w369 w382] -> w360
                tunnel: w359 -> [w368 w381]
                tunnel: [w370 w380] -> w358
                tunnel: w357 -> [w370 w379]
                tunnel: w356 -> [w366 w378]
                tunnel: w355 -> [w365 _]
                frame False {
                  n84 = Add(x=w366, y=w365) -> (x+y=w367:dbl)
                  n85 = Bundle By Name(cluster=w368, "Stop.Perm.Time Cond 2"=w367) -> (w369:T2)
                }
                frame True {
                  n86 = call "Main - Seconds to Time (SubVI).vi"("Seconds"=w378) -> ("Time string"=w375:string)  [unwired: 9 in, 1 out]
                  n87 = Bundle By Name(cluster=w381, "Stop.Perm.PostStop Run"=TRUE ("Stop.TS.PostStop Run")) -> (w382:T2)
                  n88 = Format Into String(format string="Stop Condition meet where constant flow over >= %s", initial string="", error in=w379, w375) -> (resulting string=w384:string, error out=w380:errorcluster)
                }
              }
            }
          }
        }
        frame 2 {
          n89 = Greater?(x=w393, y=w392) -> (0:w391:bool)
          n90 = case shown="True" w391 {
            tunnel: [RunTest_-_State."Check Log" RunTest_-_State."Log"] -> w396
            tunnel: ["" w409] -> w395
            tunnel: [FALSE TRUE] -> w394
            tunnel: w390 -> [w398 w408]
            tunnel: [w398 w407] -> w389
            tunnel: w388 -> [_ w405]
            tunnel: w387 -> [w397 w403]
            tunnel: [w397 w402] -> w386
            frame False {
            }
            frame True {
              n91 = call "Main - Seconds to Time (SubVI).vi"("Seconds"=w405) -> ("Time string"=w406:string)  [unwired: 9 in, 1 out]
              n92 = Bundle By Name(cluster=w403, "Stop.Perm.PostStop Run"=TRUE ("Stop.TS.PostStop Run")) -> (w402:T2)
              n93 = Format Into String(format string="Stop Condition meet where Time >= %s", initial string="", error in=w408, w406) -> (resulting string=w409:string, error out=w407:errorcluster)
            }
          }
        }
        frame 3 {
          n94 = Divide(x=w430, y=w429) -> (x/y=w426:sgl)
          n95 = Greater Or Equal?(x=w418, y=w425) -> (x >= y?=w414:bool)
          n96 = Greater?(x=w418, y=w417) -> (0:w416:bool)
          n97 = In Range and Coerce(upper limit=w428, x=w426, lower limit=w427) -> (In Range?=w424:bool)  [unwired: 1 out]
          n98 = case shown="False" w414 {
            tunnel: [w438 w471] -> w433
            tunnel: [w440 w470] -> w432
            tunnel: [w439 w469] -> w431
            tunnel: w424 -> [_ w468]
            tunnel: [w437 w467] -> w423
            tunnel: w422 -> [w436 w466]
            tunnel: [w441 w465] -> w421
            tunnel: w420 -> [w442 w464]
            tunnel: w419 -> [_ w463]
            tunnel: w418 -> [_ w462]
            tunnel: w416 -> [w434 w461]
            tunnel: w415 -> [w435 w460]
            frame False {
              n99 = case shown="True" w434 {
                tunnel: [RunTest_-_State."Check Log" RunTest_-_State."Log"] -> w438
                tunnel: ["" w455] -> w440
                tunnel: [FALSE TRUE] -> w439
                tunnel: w442 -> [w444 w454]
                tunnel: [w444 w453] -> w441
                tunnel: w435 -> [_ w451]
                tunnel: w436 -> [w443 w449]
                tunnel: [w443 w448] -> w437
                frame False {
                }
                frame True {
                  n100 = call "Main - Seconds to Time (SubVI).vi"("Seconds"=w451) -> ("Time string"=w452:string)  [unwired: 9 in, 1 out]
                  n101 = Bundle By Name(cluster=w449, "Stop.Perm.PostStop Run"=TRUE ("Stop.TS.PostStop Run")) -> (w448:T2)
                  n102 = Format Into String(format string="Stop Condition meet where Time >= %s", initial string="", error in=w454, w452) -> (resulting string=w455:string, error out=w453:errorcluster)
                }
              }
            }
            frame True {
              n103 = case shown="False" w468 {
                tunnel: [w478 RunTest_-_State."Log"] -> w471
                tunnel: [w476 w503] -> w470
                tunnel: [w477 TRUE] -> w469
                tunnel: [w479 w511] -> w467
                tunnel: w466 -> [w484 w512]
                tunnel: [w475 w504] -> w465
                tunnel: w464 -> [w474 w505]
                tunnel: w463 -> [w483 w502]
                tunnel: w462 -> [w482 _]
                tunnel: w461 -> [w473 _]
                tunnel: w460 -> [w472 _]
                frame False {
                  n104 = Add(x=w483, y=w482) -> (x+y=w481:dbl)
                  n105 = Bundle By Name(cluster=w484, "Stop.Perm.Time Cond 2"=w481) -> (w480:T2)
                  n106 = case shown="False" w473 {
                    tunnel: [RunTest_-_State."Check Log" RunTest_-_State."Log"] -> w478
                    tunnel: ["" w497] -> w476
                    tunnel: [FALSE TRUE] -> w477
                    tunnel: w474 -> [w486 w496]
                    tunnel: [w486 w495] -> w475
                    tunnel: w472 -> [_ w493]
                    tunnel: w480 -> [w485 w491]
                    tunnel: [w485 w490] -> w479
                    frame False {
                    }
                    frame True {
                      n107 = call "Main - Seconds to Time (SubVI).vi"("Seconds"=w493) -> ("Time string"=w494:string)  [unwired: 9 in, 1 out]
                      n108 = Bundle By Name(cluster=w491, "Stop.Perm.PostStop Run"=TRUE ("Stop.TS.PostStop Run")) -> (w490:T2)
                      n109 = Format Into String(format string="Stop Condition meet where Time >= %s", initial string="", error in=w496, w494) -> (resulting string=w497:string, error out=w495:errorcluster)
                    }
                  }
                }
                frame True {
                  n110 = call "Main - Seconds to Time (SubVI).vi"("Seconds"=w502) -> ("Time string"=w506:string)  [unwired: 9 in, 1 out]
                  n111 = Bundle By Name(cluster=w512, "Stop.Perm.PostStop Run"=TRUE ("Stop.TS.PostStop Run")) -> (w511:T2)
                  n112 = Format Into String(format string="Stop Condition meet where constant flow over >= %s", initial string="", error in=w505, w506) -> (resulting string=w503:string, error out=w504:errorcluster)
                }
              }
            }
          }
        }
      }
      n113 = Divide(x=w309, y=w308) -> (x/y=w307:sgl)
      n114 = Bundle(cluster=T1 {"Time Cond 2"=0.0, "Current Time"=0.0, "H Ratio"=0.0, "L Ratio"=0.0, "IF/OF"=0.0, "Ratio =1; Max=2"=0}, "Time Cond 2"=w313, "Current Time"=w312, "H Ratio"=w311, "L Ratio"=w310, "IF/OF"=w307, "Ratio =1; Max=2"=w306) -> (→"Perm":T1)
    }
    frame 5 {
      n115 = Unbundle By Name(w523) -> ("Stop.Cons.Select"=w521:i32, "Stop.Cons.Swell"=w515:bool, "Test RunTime"=w518:dbl)
      n116 = Subtract(x=w514, y=w518) -> (x-y=w520:dbl)
      n117 = Greater Or Equal?(x=w520, y=10.0) -> (x >= y?=w517:bool)
      n118 = case shown="True" w517 {
        tunnel: [w531 w550] -> w527
        tunnel: w526 -> [w531 w549]
        tunnel: [RunTest_-_State."Check Log" w548] -> w525
        tunnel: [w533 w547] -> w524
        tunnel: w523 -> [w534 w546]
        tunnel: ["" w545] -> w522
        tunnel: w521 -> [w532 w544]
        tunnel: [FALSE w543] -> w516
        tunnel: w515 -> [_ w542]
        tunnel: w514 -> [_ w541]
        frame False {
          n119 = case shown="0, Default" w532 {
            tunnel: [w539 w540] -> w533
            tunnel: w534 -> [w538 w540]
            frame 0, Default {
              n120 = Unbundle By Name(w538) -> ("Sensor Data"=w537:sgl[])
              n121 = Index Array(array=w537, index=1) -> (element=w535:sgl)
              n122 = Bundle By Name(cluster=w538, "Stop.Cons.Last Disp"=w535) -> (w539:T2)
            }
            frame 1 {
            }
          }
        }
        frame True {
          n123 = case shown="0, Default" w544 {
            tunnel: [w575 w755] -> w550
            tunnel: w549 -> [w566 w748]
            tunnel: [w569 w753] -> w548
            tunnel: [w574 w754] -> w547
            tunnel: w546 -> [w559 w742]
            tunnel: [w568 w750] -> w545
            tunnel: [w564 w747] -> w543
            tunnel: w542 -> [w558 w741]
            tunnel: w541 -> [w555 w737]
            frame 0, Default {
              n124 = Unbundle By Name(w559) -> ("Sensor Data"=w565:sgl[], "Stop.Cons.Last Disp"=w572:dbl, "Stop.Cons.Disp"=w571:dbl, "Stop.Cons.Time"=w570:dbl, "Stop.Cons.Time Cond"=w567:dbl)
              n125 = Unbundle By Name(w559) -> ("Sensor Data"=w562:sgl[], "Init.Disp Cons"=w563:sgl, "Stop.Cons.Disp 2"=w556:dbl)
              n126 = Index Array(array=w562, index=1) -> (element=w561:sgl)
              n127 = Greater Or Equal?(x=w567, y=w555) -> (x >= y?=w573:bool)
              n128 = Subtract(x=w561, y=w563) -> (x-y=w554:sgl)
              n129 = Absolute Value(x=w554) -> (abs(x)=w557:sgl)
              n130 = Less Than 0?(x=w554) -> (x < 0?=w553:bool)
              n131 = Greater?(x=w557, y=w556) -> (0:w552:bool)
              n132 = And(x=w553, y=w552) -> (x .and. y?=w551:bool)
              n133 = case shown="False" w573 {
                tunnel: [w596 w732] -> w575
                tunnel: w566 -> [w597 w732]
                tunnel: [w605 w731] -> w574
                tunnel: w559 -> [w604 w731]
                tunnel: w572 -> [w600 _]
                tunnel: w571 -> [w593 _]
                tunnel: w570 -> [w603 _]
                tunnel: w567 -> [w602 _]
                tunnel: [w606 RunTest_-_State."Check Log"] -> w569
                tunnel: w567 -> [w594 w728]
                tunnel: [w588 ""] -> w568
                tunnel: w555 -> [_ w727]
                tunnel: w565 -> [w587 _]
                tunnel: [w583 FALSE] -> w564
                tunnel: w558 -> [w582 _]
                tunnel: w551 -> [w581 _]
                tunnel: w557 -> [w580 _]
                tunnel: w556 -> [w579 _]
                frame False {
                  n134 = Add(x=w603, y=w602) -> (x+y=w601:dbl)
                  n135 = Index Array(array=w587, index=1) -> (element=w585:sgl)
                  n136 = call "Main - Seconds to Time (SubVI).vi"("Seconds"=w594) -> ("Time"=w592:timestamp)  [unwired: 9 in, 1 out]
                  n137 = Subtract(x=w585, y=w600) -> (x-y=w599:dbl)
                  n138 = Absolute Value(x=w599) -> (abs(x)=w578:dbl)
                  n139 = Format Date/Time String(time format string (%c)="%H:%M:%S", seconds (now)=w592, UTC format=FALSE) -> (date/time string=w590:string)
                  n140 = call "Main - Round Decimal Places.vi"("DecimalPlaces"=u8 3, "Number to round"=w578) -> ("Rounded number"=w577:dbl)  [unwired: 9 in]
                  n141 = Less Or Equal?(x=w577, y=w593) -> (x <= y?=w598:bool)
                  n142 = case shown="True" w582 {
                    tunnel: [w621 w667] -> w606
                    tunnel: [w620 w666] -> w605
                    tunnel: w604 -> [w619 w665]
                    tunnel: w601 -> [w618 w664]
                    tunnel: w598 -> [w617 w663]
                    tunnel: w597 -> [w616 w662]
                    tunnel: [w615 w661] -> w596
                    tunnel: "Stop Condition meet where Delta Disp (%f) <= %f. Time >= %s" -> [w614 w660]
                    tunnel: w593 -> [w613 w659]
                    tunnel: w577 -> [w612 w658]
                    tunnel: w590 -> [w611 w657]
                    tunnel: [w610 w656] -> w588
                    tunnel: w585 -> [w609 w655]
                    tunnel: "Stop Condition NOT meet where Delta Disp (%f) <= %f. Time >= %s" -> [w608 w654]
                    tunnel: [w607 w653] -> w583
                    tunnel: w581 -> [_ w652]
                    tunnel: w580 -> [_ w651]
                    tunnel: w579 -> [_ w650]
                    frame False {
                      n143 = case shown="False" w617 {
                        tunnel: [RunTest_-_State."Log" RunTest_-_State."Check Log"] -> w621
                        tunnel: [w634 w648] -> w620
                        tunnel: w619 -> [w633 w647]
                        tunnel: w618 -> [_ w646]
                        tunnel: w609 -> [_ w645]
                        tunnel: w616 -> [w631 w643]
                        tunnel: [w630 w642] -> w615
                        tunnel: w614 -> [w629 _]
                        tunnel: w613 -> [w624 w637]
                        tunnel: w612 -> [w625 w638]
                        tunnel: w611 -> [w627 w639]
                        tunnel: [w626 w641] -> w610
                        tunnel: w608 -> [_ w640]
                        tunnel: [TRUE TRUE] -> w607
                        frame True {
                          n144 = Bundle By Name(cluster=w633, "Last Log"=TRUE, "Running?"=FALSE) -> (w634:T2)
                          n145 = Format Into String(format string=w629, initial string="", error in=w631, w625, w624, w627) -> (resulting string=w626:string, error out=w630:errorcluster)
                        }
                        frame False {
                          n146 = Bundle By Name(cluster=w647, "Stop.Cons.Last Disp"=w645, "Stop.Cons.Time Cond"=w646) -> (w648:T2)
                          n147 = Format Into String(format string=w640, initial string="", error in=w643, w638, w637, w639) -> (resulting string=w641:string, error out=w642:errorcluster)
                        }
                      }
                    }
                    frame True {
                      n148 = case shown="False" w652 {
                        tunnel: [w682 RunTest_-_State."Log"] -> w667
                        tunnel: [w681 w722] -> w666
                        tunnel: w665 -> [w680 w721]
                        tunnel: w664 -> [w679 _]
                        tunnel: w663 -> [w678 _]
                        tunnel: w662 -> [w677 w720]
                        tunnel: [w676 w719] -> w661
                        tunnel: w660 -> [w675 _]
                        tunnel: w659 -> [w674 _]
                        tunnel: w658 -> [w673 _]
                        tunnel: w657 -> [w672 _]
                        tunnel: [w671 w718] -> w656
                        tunnel: w655 -> [w670 _]
                        tunnel: w654 -> [w669 _]
                        tunnel: [w668 TRUE] -> w653
                        tunnel: w651 -> [_ w713]
                        tunnel: w650 -> [_ w712]
                        frame False {
                          n149 = case shown="True" w678 {
                            tunnel: [RunTest_-_State."Log" RunTest_-_State."Check Log"] -> w682
                            tunnel: [w695 w709] -> w681
                            tunnel: w680 -> [w694 w708]
                            tunnel: w679 -> [_ w707]
                            tunnel: w670 -> [_ w706]
                            tunnel: w677 -> [w692 w704]
                            tunnel: [w691 w703] -> w676
                            tunnel: w675 -> [w690 _]
                            tunnel: w674 -> [w685 w698]
                            tunnel: w673 -> [w686 w699]
                            tunnel: w672 -> [w688 w700]
                            tunnel: [w687 w702] -> w671
                            tunnel: w669 -> [_ w701]
                            tunnel: [TRUE TRUE] -> w668
                            frame True {
                              n150 = Bundle By Name(cluster=w694, "Last Log"=TRUE, "Running?"=FALSE) -> (w695:T2)
                              n151 = Format Into String(format string=w690, initial string="", error in=w692, w686, w685, w688) -> (resulting string=w687:string, error out=w691:errorcluster)
                            }
                            frame False {
                              n152 = Bundle By Name(cluster=w708, "Stop.Cons.Last Disp"=w706, "Stop.Cons.Time Cond"=w707) -> (w709:T2)
                              n153 = Format Into String(format string=w701, initial string="", error in=w704, w699, w698, w700) -> (resulting string=w702:string, error out=w703:errorcluster)
                            }
                          }
                        }
                        frame True {
                          n154 = Bundle By Name(cluster=w721, "Last Log"=TRUE, "Running?"=FALSE) -> (w722:T2)
                          n155 = Format Into String(format string="Stop Condition meet where %f <= Delta Disp (%f).", initial string="", error in=w720, w712, w713) -> (resulting string=w718:string, error out=w719:errorcluster)
                        }
                      }
                    }
                  }
                }
                frame True {
                  n156 = Subtract(x=w728, y=w727) -> (x-y=w726:dbl)
                  n157 = call "Main - Seconds to Time (SubVI).vi"("Seconds"=w726) -> ("Time string"=w724:string)  [unwired: 9 in, 1 out]
                  n158 = local write "Delay"(w724) -> ()
                }
              }
            }
            frame 1 {
              n159 = Unbundle By Name(w742) -> ("Sensor Data"=w745:sgl[], "Init.Disp Cons"=w746:sgl, "Stop.Cons.Disp 2"=w739:dbl)
              n160 = Unbundle By Name(w742) -> ("Stop.Cons.Time2"=w751:dbl, "Stop.Cons.Time Cond"=w752:dbl)
              n161 = Index Array(array=w745, index=1) -> (element=w744:sgl)
              n162 = Subtract(x=w737, y=w752) -> (x-y=w749:dbl)
              n163 = Subtract(x=w744, y=w746) -> (x-y=w734:sgl)
              n164 = Greater?(x=w749, y=w751) -> (0:w740:bool)
              n165 = Absolute Value(x=w734) -> (abs(x)=w738:sgl)
              n166 = Less Than 0?(x=w734) -> (x < 0?=w733:bool)
              n167 = Greater?(x=w738, y=w739) -> (0:w736:bool)
              n168 = And(x=w733, y=w736) -> (x .and. y?=w735:bool)
              n169 = case shown="False" w741 {
                tunnel: [w765 w800] -> w755
                tunnel: [w764 w799] -> w754
                tunnel: [w763 w798] -> w753
                tunnel: w751 -> [w762 w797]
                tunnel: [w761 w796] -> w750
                tunnel: w749 -> [w760 w795]
                tunnel: w748 -> [w759 w794]
                tunnel: [w758 w793] -> w747
                tunnel: w742 -> [w757 w792]
                tunnel: w740 -> [w756 w791]
                tunnel: w735 -> [_ w790]
                tunnel: w739 -> [_ w789]
                tunnel: w738 -> [_ w788]
                frame False {
                  n170 = case shown="True" w756 {
                    tunnel: [w774 w781] -> w765
                    tunnel: w759 -> [w774 w780]
                    tunnel: [w773 w786] -> w764
                    tunnel: w757 -> [w773 w785]
                    tunnel: [RunTest_-_State."Check Log" RunTest_-_State."Log"] -> w763
                    tunnel: w762 -> [w770 w779]
                    tunnel: ["" w778] -> w761
                    tunnel: w760 -> [w769 _]
                    tunnel: [FALSE TRUE] -> w758
                    frame False {
                      n171 = Subtract(x=w770, y=w769) -> (x-y=w768:dbl)
                      n172 = call "Main - Seconds to Time (SubVI).vi"("Seconds"=w768) -> ("Time string"=w766:string)  [unwired: 9 in, 1 out]
                      n173 = local write "Delay"(w766) -> ()
                    }
                    frame True {
                      n174 = call "Main - Seconds to Time (SubVI).vi"("Seconds"=w779) -> ("Time string"=w776:string)  [unwired: 9 in, 1 out]
                      n175 = Bundle By Name(cluster=w785, "Last Log"=TRUE, "Running?"=FALSE) -> (w786:T2)
                      n176 = Format Into String(format string="Stop Condition meet where Time >= %s", initial string="", error in=w780, w776) -> (resulting string=w778:string, error out=w781:errorcluster)
                    }
                  }
                }
                frame True {
                  n177 = case shown="False" w790 {
                    tunnel: [w810 w845] -> w800
                    tunnel: [w809 w844] -> w799
                    tunnel: [w808 RunTest_-_State."Log"] -> w798
                    tunnel: w797 -> [w807 _]
                    tunnel: [w806 w842] -> w796
                    tunnel: w795 -> [w805 _]
                    tunnel: w794 -> [w804 w841]
                    tunnel: [w803 TRUE] -> w793
                    tunnel: w792 -> [w802 w839]
                    tunnel: w791 -> [w801 _]
                    tunnel: w789 -> [_ w838]
                    tunnel: w788 -> [_ w837]
                    frame False {
                      n178 = case shown="True" w801 {
                        tunnel: [w819 w826] -> w810
                        tunnel: w804 -> [w819 w825]
                        tunnel: [w818 w831] -> w809
                        tunnel: w802 -> [w818 w830]
                        tunnel: [RunTest_-_State."Check Log" RunTest_-_State."Log"] -> w808
                        tunnel: w807 -> [w815 w824]
                        tunnel: ["" w823] -> w806
                        tunnel: w805 -> [w814 _]
                        tunnel: [FALSE TRUE] -> w803
                        frame False {
                          n179 = Subtract(x=w815, y=w814) -> (x-y=w813:dbl)
                          n180 = call "Main - Seconds to Time (SubVI).vi"("Seconds"=w813) -> ("Time string"=w811:string)  [unwired: 9 in, 1 out]
                          n181 = local write "Delay"(w811) -> ()
                        }
                        frame True {
                          n182 = call "Main - Seconds to Time (SubVI).vi"("Seconds"=w824) -> ("Time string"=w821:string)  [unwired: 9 in, 1 out]
                          n183 = Bundle By Name(cluster=w830, "Last Log"=TRUE, "Running?"=FALSE) -> (w831:T2)
                          n184 = Format Into String(format string="Stop Condition meet where Time >= %s", initial string="", error in=w825, w821) -> (resulting string=w823:string, error out=w826:errorcluster)
                        }
                      }
                    }
                    frame True {
                      n185 = Bundle By Name(cluster=w839, "Last Log"=TRUE, "Running?"=FALSE) -> (w844:T2)
                      n186 = Format Into String(format string="Stop Condition meet where %f <= Delta Disp (%f).", initial string="", error in=w841, w838, w837) -> (resulting string=w842:string, error out=w845:errorcluster)
                    }
                  }
                }
              }
            }
          }
        }
      }
    }
    frame 6 {
      # "Cp\nBP\nVC\nPP\nB-Value"
      n187 = Unbundle By Name(w858) -> ("Stop.Sat.Select"=w846:i32, "Sensor Data"=w850:sgl[], "Stop.Sat..B"=w854:bool, "Stop.Sat.B"=w849:dbl, "Test RunTime"=w847:dbl)
      n188 = Index Array(array=w850, index=4) -> (element=w848:sgl)
      n189 = Greater Or Equal?(x=w848, y=w849) -> (x >= y?=w853:bool)
      n190 = And(x=w854, y=w853) -> (x .and. y?=w852:bool)
      n191 = case shown="False" w852 {
        tunnel: [w872 w1064] -> w862
        tunnel: w861 -> [w871 w1065]
        tunnel: [w867 w1071] -> w859
        tunnel: w858 -> [w868 w1068]
        tunnel: [w866 RunTest_-_State."Log"] -> w860
        tunnel: w849 -> [_ w1063]
        tunnel: w848 -> [_ w1062]
        tunnel: [w865 w1061] -> w857
        tunnel: [w864 TRUE] -> w856
        tunnel: w855 -> [w870 w1058]
        tunnel: w847 -> [w869 _]
        tunnel: w846 -> [w863 _]
        frame False {
          n192 = case shown="7" w863 {
            tunnel: [w874 w888 w897 w916 w939 w958 w991 w1029] -> w872
            tunnel: w871 -> [w874 w887 w898 w910 w940 w954 w981 w1012]
            tunnel: w870 -> [_ w886 w890 w912 w932 w951 w975 w1010]
            tunnel: w869 -> [_ w885 w889 w913 _ w950 w974 w1011]
            tunnel: w868 -> [w878 w884 w891 w908 w933 w952 w982 w1015]
            tunnel: [w878 w883 w893 w914 w935 w956 w989 w1027] -> w867
            tunnel: [RunTest_-_State."Idle" ("Enum") w882 w892 w907 w934 w943 w985 w1023] -> w866
            tunnel: ["" ("Event") w881 w895 w906 w937 w941 w983 w1021] -> w865
            tunnel: [FALSE ("Boolean") w880 w894 w904 w936 w942 w984 w1022] -> w864
            tunnel: ["" ("Time string") w879 w896 w915 w938 w957 w990 w1028] -> _
            frame 0, Default {
            }
            frame 1 {
              n193 = call "Stop Condition - Saturation 1 (SubVI).vi"("error in (no error)"=w887, "Test RunTime"=w885, "Time"=w886, "Cluster in"=w884) -> ("error out"=w888:errorcluster, "Event"=w881:string, "Boolean"=w880:bool, "Cluster out"=w883:T2, "Delay"=w879:string, "Enum"=w882:T11)  [unwired: 2 in]
            }
            frame 2 {
              n194 = call "Stop Condition - Saturation 2 (SubVI).vi"("error in (no error)"=w898, "Test RunTime"=w889, "Time"=w890, "Cluster in"=w891) -> ("error out"=w897:errorcluster, "String"=w895:string, "Boolean"=w894:bool, "Cluster out"=w893:T2, "Delay"=w896:string, "Enum"=w892:T11)  [unwired: 2 in]
            }
            frame 3 {
              n195 = call "Stop Condition - Saturation 1 (SubVI).vi"("error in (no error)"=w910, "Test RunTime"=w913, "Time"=w912, "Cluster in"=w908) -> ("error out"=w911:errorcluster, "Event"=w905:string, "Boolean"=w899:bool, "Cluster out"=w909:T2, "Enum"=w900:T11)  [unwired: 2 in, 1 out]
              n196 = call "Stop Condition - Saturation 2 (SubVI).vi"("error in (no error)"=w911, "Test RunTime"=w913, "Time"=w912, "Cluster in"=w909) -> ("error out"=w916:errorcluster, "String"=w901:string, "Boolean"=w903:bool, "Cluster out"=w914:T2, "Delay"=w915:string, "Enum"=w902:T11)  [unwired: 2 in]
              n197 = case shown="Default" w900 {
                selector: w900 -> [_ w930]
                tunnel: [w919 w930] -> w907
                tunnel: [w921 w931] -> w906
                tunnel: w905 -> [_ w931]
                tunnel: [w920 w929] -> w904
                tunnel: w903 -> [w917 _]
                tunnel: w902 -> [w918 _]
                tunnel: w901 -> [w922 _]
                tunnel: w899 -> [_ w929]
                frame Default {
                  n198 = case shown="Default" w918 {
                    selector: w918 -> [w925 w927]
                    tunnel: w922 -> [w923 w928]
                    tunnel: [w923 w928] -> w921
                    tunnel: [w924 w926] -> w920
                    tunnel: [w925 w927] -> w919
                    tunnel: w917 -> [w924 w926]
                    frame "Log" {
                    }
                    frame Default {
                    }
                  }
                }
                frame "Log" {
                }
              }
            }
            frame 4 {
              n199 = call "Stop Condition - Saturation 4 (SubVI).vi"("error in (no error)"=w940, "Time"=w932, "Cluster in"=w933) -> ("error out"=w939:errorcluster, "String"=w937:string, "Boolean"=w936:bool, "Cluster out"=w935:T2, "Delay"=w938:string, "Enum"=w934:T11)  [unwired: 3 in]
            }
            frame 5 {
              n200 = call "Stop Condition - Saturation 1 (SubVI).vi"("error in (no error)"=w954, "Test RunTime"=w950, "Time"=w951, "Cluster in"=w952) -> ("error out"=w955:errorcluster, "Event"=w947:string, "Boolean"=w948:bool, "Cluster out"=w953:T2, "Enum"=w949:T11)  [unwired: 2 in, 1 out]
              n201 = call "Stop Condition - Saturation 4 (SubVI).vi"("error in (no error)"=w955, "Time"=w951, "Cluster in"=w953) -> ("error out"=w958:errorcluster, "String"=w944:string, "Boolean"=w945:bool, "Cluster out"=w956:T2, "Delay"=w957:string, "Enum"=w946:T11)  [unwired: 3 in]
              n202 = case shown="Default" w949 {
                selector: w949 -> [_ w972]
                tunnel: [w961 w972] -> w943
                tunnel: [w963 w973] -> w941
                tunnel: w947 -> [_ w973]
                tunnel: [w962 w971] -> w942
                tunnel: w945 -> [w959 _]
                tunnel: w946 -> [w960 _]
                tunnel: w944 -> [w964 _]
                tunnel: w948 -> [_ w971]
                frame Default {
                  n203 = case shown="Default" w960 {
                    selector: w960 -> [w967 w969]
                    tunnel: w964 -> [w965 w970]
                    tunnel: [w965 w970] -> w963
                    tunnel: [w966 w968] -> w962
                    tunnel: [w967 w969] -> w961
                    tunnel: w959 -> [w966 w968]
                    frame "Log" {
                    }
                    frame Default {
                    }
                  }
                }
                frame "Log" {
                }
              }
            }
            frame 6 {
              n204 = call "Stop Condition - Saturation 2 (SubVI).vi"("error in (no error)"=w981, "Test RunTime"=w974, "Time"=w975, "Cluster in"=w982) -> ("error out"=w980:errorcluster, "String"=w979:string, "Boolean"=w978:bool, "Cluster out"=w976:T2, "Enum"=w977:T11)  [unwired: 2 in, 1 out]
              n205 = call "Stop Condition - Saturation 4 (SubVI).vi"("error in (no error)"=w980, "Time"=w975, "Cluster in"=w976) -> ("error out"=w991:errorcluster, "String"=w986:string, "Boolean"=w987:bool, "Cluster out"=w989:T2, "Delay"=w990:string, "Enum"=w988:T11)  [unwired: 3 in]
              n206 = case shown="Default" w977 {
                selector: w977 -> [_ w1005]
                tunnel: [w994 w1005] -> w985
                tunnel: [w996 w1006] -> w983
                tunnel: w979 -> [_ w1006]
                tunnel: [w995 w1004] -> w984
                tunnel: w987 -> [w992 _]
                tunnel: w988 -> [w993 _]
                tunnel: w986 -> [w997 _]
                tunnel: w978 -> [_ w1004]
                frame Default {
                  n207 = case shown="Default" w993 {
                    selector: w993 -> [w1000 w1002]
                    tunnel: w997 -> [w998 w1003]
                    tunnel: [w998 w1003] -> w996
                    tunnel: [w999 w1001] -> w995
                    tunnel: [w1000 w1002] -> w994
                    tunnel: w992 -> [w999 w1001]
                    frame "Log" {
                    }
                    frame Default {
                    }
                  }
                }
                frame "Log" {
                }
              }
            }
            frame 7 {
              n208 = call "Stop Condition - Saturation 1 (SubVI).vi"("error in (no error)"=w1012, "Test RunTime"=w1011, "Time"=w1010, "Cluster in"=w1015) -> ("error out"=w1013:errorcluster, "Event"=w1007:string, "Boolean"=w1008:bool, "Cluster out"=w1014:T2, "Enum"=w1009:T11)  [unwired: 2 in, 1 out]
              n209 = call "Stop Condition - Saturation 2 (SubVI).vi"("error in (no error)"=w1013, "Test RunTime"=w1011, "Time"=w1010, "Cluster in"=w1014) -> ("error out"=w1020:errorcluster, "String"=w1019:string, "Boolean"=w1018:bool, "Cluster out"=w1016:T2, "Enum"=w1017:T11)  [unwired: 2 in, 1 out]
              n210 = call "Stop Condition - Saturation 4 (SubVI).vi"("error in (no error)"=w1020, "Time"=w1010, "Cluster in"=w1016) -> ("error out"=w1029:errorcluster, "String"=w1024:string, "Boolean"=w1025:bool, "Cluster out"=w1027:T2, "Delay"=w1028:string, "Enum"=w1026:T11)  [unwired: 3 in]
              n211 = case shown="Default" w1009 {
                selector: w1009 -> [w1032 _]
                tunnel: w1026 -> [_ w1041]
                tunnel: w1025 -> [_ w1040]
                tunnel: w1024 -> [_ w1039]
                tunnel: [w1032 w1038] -> w1023
                tunnel: [w1031 w1037] -> w1022
                tunnel: [w1030 w1036] -> w1021
                tunnel: w1019 -> [_ w1035]
                tunnel: w1018 -> [_ w1034]
                tunnel: w1017 -> [_ w1033]
                tunnel: w1008 -> [w1031 _]
                tunnel: w1007 -> [w1030 _]
                frame "Log" {
                }
                frame Default {
                  n212 = case shown="Default" w1033 {
                    selector: w1033 -> [_ w1055]
                    tunnel: [w1044 w1055] -> w1038
                    tunnel: [w1046 w1056] -> w1036
                    tunnel: w1035 -> [_ w1056]
                    tunnel: [w1045 w1054] -> w1037
                    tunnel: w1040 -> [w1042 _]
                    tunnel: w1041 -> [w1043 _]
                    tunnel: w1039 -> [w1047 _]
                    tunnel: w1034 -> [_ w1054]
                    frame Default {
                      n213 = case shown="Default" w1043 {
                        selector: w1043 -> [w1050 w1052]
                        tunnel: w1047 -> [w1048 w1053]
                        tunnel: [w1048 w1053] -> w1046
                        tunnel: [w1049 w1051] -> w1045
                        tunnel: [w1050 w1052] -> w1044
                        tunnel: w1042 -> [w1049 w1051]
                        frame "Log" {
                        }
                        frame Default {
                        }
                      }
                    }
                    frame "Log" {
                    }
                  }
                }
              }
            }
          }
        }
        frame True {
          n214 = call "Main - Seconds to Time (SubVI).vi"("Seconds"=w1058) -> ("Time string"=w1059:string)  [unwired: 9 in, 1 out]
          n215 = Bundle By Name(cluster=w1068, "Stop.Sat.B Achieve"=TRUE, "Running?"=FALSE) -> (w1071:T2)
          n216 = Format Into String(format string="Stop Condition meet where B-Value (%f) > %f. Time = %s", initial string="", error in=w1065, w1062, w1063, w1059) -> (resulting string=w1061:string, error out=w1064:errorcluster)
        }
      }
    }
    frame 8 {
      (unwired) string[] ["Cell Pressure", "Back Pressure", "Volume Change", "Load", "Displacement", "Pore Pressure", "Change of Pore Pressure", "Change in Volume", "Axial Load Change", "Change in Length", "Deviator Stress", "Axial Strain"]  # Triaxial Shear
      n217 = Unbundle By Name(w1082) -> ("Stop.UCT.MaxDev Value"=w1073:dbl, "Stop.UCT..MaxDev"=w1075:bool, "Calc.UCT.Axial Strain"=w1076:sgl, "Stop.UCT.Axial"=w1077:dbl)
      n218 = Greater?(x=w1076, y=w1077) -> (0:w1084:bool)
      n219 = case shown="True" w1084 {
        tunnel: [w1091 w1156] -> w1083
        tunnel: w1082 -> [w1090 w1155]
        tunnel: [w1093 w1165] -> w1081
        tunnel: w1080 -> [w1092 w1164]
        tunnel: [w1086 w1162] -> w1079
        tunnel: [w1088 TRUE] -> w1078
        tunnel: w1077 -> [_ w1160]
        tunnel: w1076 -> [_ w1159]
        tunnel: w1075 -> [w1094 _]
        tunnel: [w1089 RunTest_-_State."Log"] -> w1074
        tunnel: w1073 -> [w1087 _]
        tunnel: w1072 -> [w1085 _]
        frame False {
          n220 = case shown="True" w1094 {
            tunnel: [w1098 w1106] -> w1093
            tunnel: w1092 -> [w1098 w1105]
            tunnel: [w1095 w1108] -> w1091
            tunnel: w1090 -> [w1095 w1107]
            tunnel: [RunTest_-_State."Check Log" w1104] -> w1089
            tunnel: [FALSE w1103] -> w1088
            tunnel: w1087 -> [_ w1101]
            tunnel: [_ w1100] -> w1086
            tunnel: w1085 -> [_ w1099]
            frame False {
            }
            frame True {
              n221 = Unbundle By Name(w1107) -> ("Stop.UCT.Prev Time"=w1112:dbl, "Calc.UCT.MaxDeviator"=w1102:sgl)
              n222 = Subtract(x=w1099, y=w1112) -> (x-y=w1111:dbl)
              n223 = Greater Or Equal?(x=w1111, y=1.0) -> (x >= y?=w1109:bool)
              n224 = case shown="True" w1109 {
                tunnel: [w1115 w1133] -> w1108
                tunnel: w1107 -> [w1115 w1132]
                tunnel: [w1114 w1129] -> w1106
                tunnel: w1105 -> [w1114 w1128]
                tunnel: [RunTest_-_State."Check Log" w1131] -> w1104
                tunnel: [FALSE w1130] -> w1103
                tunnel: w1102 -> [_ w1117]
                tunnel: w1101 -> [_ w1120]
                tunnel: [_ w1119] -> w1100
                frame False {
                }
                frame True {
                  n225 = Unbundle By Name(w1132) -> ("Calc.UCT.Deviator"=w1127:sgl)
                  n226 = Subtract(x=w1117, y=w1127) -> (x-y=w1126:sgl)
                  n227 = Less?(x=w1127, y=w1117) -> (x < y?=w1123:bool)
                  n228 = Divide(x=w1126, y=w1117) -> (x/y=w1125:sgl)
                  n229 = Multiply(x=w1125, y=sgl 100.0) -> (x*y=w1118:sgl)
                  n230 = Greater?(x=w1118, y=w1120) -> (0:w1122:bool)
                  n231 = And(x=w1123, y=w1122) -> (x .and. y?=w1121:bool)
                  n232 = case shown="False" w1121 {
                    tunnel: [w1139 w1144] -> w1133
                    tunnel: w1132 -> [w1138 w1143]
                    tunnel: [RunTest_-_State."Check Log" RunTest_-_State."Log"] -> w1131
                    tunnel: [FALSE TRUE] -> w1130
                    tunnel: [w1140 w1149] -> w1129
                    tunnel: w1128 -> [w1140 w1150]
                    tunnel: w1118 -> [_ w1148]
                    tunnel: w1120 -> [_ w1147]
                    tunnel: [_ w1146] -> w1119
                    frame False {
                      n233 = Unbundle By Name(w1138) -> ("Calc.UCT.Deviator"=w1136:sgl, "Calc.UCT.MaxDeviator"=w1135:sgl)
                      n234 = Greater?(x=w1136, y=w1135) -> (0:w1137:bool)
                      n235 = Select(t=w1136, s=w1137, f=w1135) -> (s? t:f=w1134:sgl)
                      n236 = Bundle By Name(cluster=w1138, "Calc.UCT.MaxDeviator"=w1134) -> (w1139:T2)
                    }
                    frame True {
                      n237 = Bundle By Name(cluster=w1143, "Stop.UCT.PostStop Run"=TRUE ("Stop.TS.PostStop Run")) -> (w1144:T2)
                      n238 = Format Into String(format string="Stop Condition meet where Max Deviator (%f) > %f", initial string="", error in=w1150, w1148, w1147) -> (resulting string=w1146:string, error out=w1149:errorcluster)
                    }
                  }
                }
              }
            }
          }
        }
        frame True {
          n239 = Bundle By Name(cluster=w1155, "Stop.UCT.PostStop Run"=TRUE ("Stop.TS.PostStop Run")) -> (w1156:T2)
          n240 = Format Into String(format string="Stop Condition meet where Axial Strain (%f) > %f", initial string="", error in=w1164, w1159, w1160) -> (resulting string=w1162:string, error out=w1165:errorcluster)
        }
      }
    }
    frame 9 {
      # "CP\nPP\nVC\nBP\nCPP\nPP Diss\nCiV"
      n241 = Unbundle By Name(w1176) -> ("Stop.Iso..PP"=w1175:bool, "Stop.Iso.Select"=w1172:i32)
      n242 = Equal To 0?(x=w1172) -> (x = 0?=w1171:bool)
      n243 = Not Equal To 0?(x=w1172) -> (x != 0?=w1170:bool)
      n244 = Build Array(w1175, w1171, w1170) -> (w1174:bool[])
      n245 = Boolean Array To Number(Boolean array=w1174) -> (number=w1173:u32)
      n246 = case shown="0, Default" w1173 {
        tunnel: [w1183 w1202 w1241 w1277 w1342] -> w1180
        tunnel: w1179 -> [w1183 w1196 w1232 w1272 w1337]
        tunnel: [RunTest_-_State."Check Log" w1199 w1238 w1274 w1339] -> w1178
        tunnel: [w1185 w1201 w1240 w1276 w1341] -> w1177
        tunnel: w1176 -> [w1185 w1200 w1239 w1275 w1340]
        tunnel: ["" ("initial string") w1189 w1228 w1265 w1331] -> w1169
        tunnel: [FALSE w1188 w1229 w1266 w1332] -> w1168
        tunnel: w1167 -> [_ w1186 w1219 w1261 w1323]
        frame 0, Default {
        }
        frame 2 {
          n247 = Unbundle By Name(w1200) -> ("Stop.Iso.Time"=w1187:dbl, "Stop.Iso.Time Cond"=w1197:dbl)
          n248 = Subtract(x=w1186, y=w1197) -> (x-y=w1191:dbl)
          n249 = Greater Or Equal?(x=w1191, y=w1187) -> (x >= y?=w1198:bool)
          n250 = call "Main - Seconds to Time (SubVI).vi"("Seconds"=w1187) -> ("Time"=w1194:timestamp)  [unwired: 9 in, 1 out]
          n251 = Format Date/Time String(time format string (%c)="%H:%M:%S", seconds (now)=w1194, UTC format=FALSE) -> (date/time string=w1190:string)
          n252 = case shown="True" w1198 {
            tunnel: [w1207 w1213] -> w1202
            tunnel: w1196 -> [w1207 w1212]
            tunnel: [w1205 w1218] -> w1201
            tunnel: w1200 -> [w1205 w1215]
            tunnel: [RunTest_-_State."Check Log" RunTest_-_State."Log"] -> w1199
            tunnel: "Stop Condition meet where Time >= %s" -> [_ w1211]
            tunnel: w1190 -> [_ w1210]
            tunnel: ["" w1209] -> w1189
            tunnel: [FALSE TRUE] -> w1188
            frame False {
            }
            frame True {
              n253 = Bundle By Name(cluster=w1215, "Running?"=FALSE) -> (w1218:T2)
              n254 = Format Into String(format string=w1211, initial string="", error in=w1212, w1210) -> (resulting string=w1209:string, error out=w1213:errorcluster)
            }
          }
        }
        frame 3 {
          n255 = Unbundle By Name(w1239) -> ("Sensor Data"=w1230:sgl[], "Stop.Iso.PP"=w1220:dbl, "Stop.Iso.Time"=w1223:dbl, "Stop.Iso.Time Cond"=w1237:dbl)
          n256 = Subtract(x=w1219, y=w1237) -> (x-y=w1236:dbl)
          n257 = Index Array(array=w1230, index=5) -> (element=w1221:sgl)
          n258 = Greater Or Equal?(x=w1221, y=w1220) -> (x >= y?=w1234:bool)
          n259 = Greater Or Equal?(x=w1236, y=w1223) -> (x >= y?=w1235:bool)
          n260 = Or(x=w1234, y=w1235) -> (x .or. y?=w1233:bool)
          n261 = call "Main - Seconds to Time (SubVI).vi"("Seconds"=w1223) -> ("Time"=w1226:timestamp)  [unwired: 9 in, 1 out]
          n262 = Format Date/Time String(time format string (%c)="%H:%M:%S", seconds (now)=w1226, UTC format=FALSE) -> (date/time string=w1222:string)
          n263 = case shown="True" w1233 {
            tunnel: [w1246 w1252] -> w1241
            tunnel: w1232 -> [w1246 w1253]
            tunnel: [w1244 w1259] -> w1240
            tunnel: w1239 -> [w1244 w1256]
            tunnel: [RunTest_-_State."Check Log" RunTest_-_State."Log"] -> w1238
            tunnel: [FALSE TRUE] -> w1229
            tunnel: ["" w1250] -> w1228
            tunnel: "Stop Condition meet where PWP Diss (%f) >= %f or Time >= %s" -> [_ w1251]
            tunnel: w1222 -> [_ w1249]
            tunnel: w1221 -> [_ w1248]
            tunnel: w1220 -> [_ w1247]
            frame False {
            }
            frame True {
              n264 = Bundle By Name(cluster=w1256, "Running?"=FALSE) -> (w1259:T2)
              n265 = Format Into String(format string=w1251, initial string="", error in=w1253, w1248, w1247, w1249) -> (resulting string=w1250:string, error out=w1252:errorcluster)
            }
          }
        }
        frame 4 {
          n266 = Unbundle By Name(w1275) -> ("Sensor Data"=w1269:sgl[], "Stop.Iso.VC"=w1263:dbl, "Stop.Iso.Time2"=w1273:dbl, "Stop.Iso.Time Cond 2"=w1262:dbl)
          n267 = Index Array(array=w1269, index #1=5 ("index"), index #2=6 ("index")) -> (element #2=w1264:sgl)  [unwired: 1 out]
          n268 = call "Main - Seconds to Time (SubVI).vi"("Seconds"=w1262) -> ("Time string"=w1260:string)  [unwired: 9 in, 1 out]
          n269 = Greater Or Equal?(x=w1262, y=w1261) -> (x >= y?=w1267:bool)
          n270 = Less Or Equal?(x=w1264, y=w1263) -> (x <= y?=w1268:bool)
          n271 = case shown="False" w1267 {
            tunnel: [w1290 w1319] -> w1277
            tunnel: [w1289 w1318] -> w1276
            tunnel: w1275 -> [w1288 w1318]
            tunnel: [w1287 RunTest_-_State."Check Log"] -> w1274
            tunnel: w1273 -> [w1286 _]
            tunnel: w1262 -> [w1285 w1317]
            tunnel: w1272 -> [w1284 w1319]
            tunnel: w1268 -> [w1283 _]
            tunnel: w1261 -> [_ w1316]
            tunnel: [w1282 FALSE] -> w1266
            tunnel: [w1281 "" ("initial string")] -> w1265
            tunnel: w1264 -> [w1280 _]
            tunnel: w1263 -> [w1279 _]
            tunnel: w1260 -> [w1278 _]
            frame False {
              n272 = case shown="True" w1283 {
                tunnel: [w1299 w1305] -> w1290
                tunnel: w1284 -> [w1299 w1306]
                tunnel: [w1297 w1312] -> w1289
                tunnel: w1288 -> [w1296 w1309]
                tunnel: [RunTest_-_State."Check Log" RunTest_-_State."Log"] -> w1287
                tunnel: w1286 -> [w1295 _]
                tunnel: w1285 -> [w1294 _]
                tunnel: [FALSE TRUE] -> w1282
                tunnel: ["" ("initial string") w1304] -> w1281
                tunnel: w1280 -> [_ w1303]
                tunnel: w1279 -> [_ w1302]
                tunnel: w1278 -> [_ w1300]
                frame False {
                  n273 = Add(x=w1295, y=w1294) -> (x+y=w1293:dbl)
                  n274 = Bundle By Name(cluster=w1296, "Stop.Iso.Time Cond 2"=w1293) -> (w1297:T2)
                }
                frame True {
                  n275 = Bundle By Name(cluster=w1309, "Running?"=FALSE) -> (w1312:T2)
                  n276 = Format Into String(format string="Stop Condition meet where Volume Change (%f) <= %f. Time >= %s", initial string="", error in=w1306, w1303, w1302, w1300) -> (resulting string=w1304:string, error out=w1305:errorcluster)
                }
              }
            }
            frame True {
              n277 = Subtract(x=w1317, y=w1316) -> (x-y=w1321:dbl)
              n278 = call "Main - Seconds to Time (SubVI).vi"("Seconds"=w1321) -> ("Time string"=w1313:string)  [unwired: 9 in, 1 out]
              n279 = local write "Delay"(w1313) -> ()
            }
          }
        }
        frame 5 {
          n280 = Unbundle By Name(w1340) -> ("Sensor Data"=w1334:sgl[], "Stop.Iso.PP"=w1324:dbl, "Stop.Iso.VC"=w1327:dbl, "Stop.Iso.Time2"=w1338:dbl, "Stop.Iso.Time Cond 2"=w1329:dbl)
          n281 = Index Array(array=w1334, index #1=5 ("index"), index #2=6 ("index")) -> (element #1=w1325:sgl, element #2=w1328:sgl)
          n282 = Greater Or Equal?(x=w1329, y=w1323) -> (x >= y?=w1333:bool)
          n283 = Less Or Equal?(x=w1328, y=w1327) -> (x <= y?=w1330:bool)
          n284 = call "Main - Seconds to Time (SubVI).vi"("Seconds"=w1329) -> ("Time string"=w1322:string)  [unwired: 9 in, 1 out]
          n285 = Greater Or Equal?(x=w1325, y=w1324) -> (x >= y?=w1326:bool)
          n286 = case shown="False" w1326 {
            tunnel: [w1357 w1406] -> w1342
            tunnel: [w1356 w1411] -> w1341
            tunnel: w1340 -> [w1355 w1412]
            tunnel: [w1354 RunTest_-_State."Log"] -> w1339
            tunnel: w1338 -> [w1353 _]
            tunnel: w1337 -> [w1352 w1407]
            tunnel: w1333 -> [w1351 _]
            tunnel: w1323 -> [w1350 _]
            tunnel: [w1349 TRUE] -> w1332
            tunnel: [w1348 w1405] -> w1331
            tunnel: w1330 -> [w1347 _]
            tunnel: w1329 -> [w1346 _]
            tunnel: w1322 -> [w1345 _]
            tunnel: w1328 -> [w1344 _]
            tunnel: w1327 -> [w1343 _]
            tunnel: w1325 -> [_ w1403]
            tunnel: w1324 -> [_ w1402]
            frame False {
              n287 = case shown="False" w1351 {
                tunnel: [w1370 w1398] -> w1357
                tunnel: [w1369 w1396] -> w1356
                tunnel: w1355 -> [w1368 w1396]
                tunnel: [w1367 RunTest_-_State."Check Log"] -> w1354
                tunnel: w1353 -> [w1366 _]
                tunnel: w1346 -> [w1365 w1400]
                tunnel: w1352 -> [w1364 w1398]
                tunnel: w1350 -> [_ w1399]
                tunnel: [w1363 FALSE] -> w1349
                tunnel: [w1362 "" ("initial string")] -> w1348
                tunnel: w1347 -> [w1361 _]
                tunnel: w1345 -> [w1360 _]
                tunnel: w1344 -> [w1359 _]
                tunnel: w1343 -> [w1358 _]
                frame False {
                  n288 = case shown="True" w1361 {
                    tunnel: [w1379 w1385] -> w1370
                    tunnel: w1364 -> [w1379 w1386]
                    tunnel: [w1377 w1392] -> w1369
                    tunnel: w1368 -> [w1376 w1389]
                    tunnel: [RunTest_-_State."Check Log" RunTest_-_State."Log"] -> w1367
                    tunnel: w1366 -> [w1375 _]
                    tunnel: w1365 -> [w1374 _]
                    tunnel: [FALSE TRUE] -> w1363
                    tunnel: ["" ("initial string") w1384] -> w1362
                    tunnel: w1360 -> [_ w1382]
                    tunnel: w1359 -> [_ w1381]
                    tunnel: w1358 -> [_ w1380]
                    frame False {
                      n289 = Add(x=w1375, y=w1374) -> (x+y=w1373:dbl)
                      n290 = Bundle By Name(cluster=w1376, "Stop.Iso.Time Cond 2"=w1373) -> (w1377:T2)
                    }
                    frame True {
                      n291 = Bundle By Name(cluster=w1389, "Running?"=FALSE) -> (w1392:T2)
                      n292 = Format Into String(format string="Stop Condition meet where Volume Change (%f) <= %f. Time >= %s", initial string="", error in=w1386, w1381, w1380, w1382) -> (resulting string=w1384:string, error out=w1385:errorcluster)
                    }
                  }
                }
                frame True {
                  n293 = Subtract(x=w1400, y=w1399) -> (x-y=w1401:dbl)
                  n294 = call "Main - Seconds to Time (SubVI).vi"("Seconds"=w1401) -> ("Time string"=w1393:string)  [unwired: 9 in, 1 out]
                  n295 = local write "Delay"(w1393) -> ()
                }
              }
            }
            frame True {
              n296 = Bundle By Name(cluster=w1412, "Running?"=FALSE) -> (w1411:T2)
              n297 = Format Into String(format string="Stop Condition meet where PWP Diss (%f) >= %f.", initial string="", error in=w1407, w1403, w1402) -> (resulting string=w1405:string, error out=w1406:errorcluster)
            }
          }
        }
      }
    }
    frame 10 {
      # "VLoad\nVStress"
      n298 = Unbundle By Name(w1421) -> ("Stop.SP..Max Time"=w1417:bool, "Stop.SP..Time"=w1414:bool)
      n299 = Build Array(w1417, w1414) -> (w1416:bool[])
      n300 = Boolean Array To Number(Boolean array=w1416) -> (number=w1415:u32)
      n301 = case shown="2" w1415 {
        tunnel: [w1428 w1444 w1476 w1532] -> w1425
        tunnel: w1424 -> [w1428 w1438 w1470 w1526]
        tunnel: [RunTest_-_State."Check Log" w1441 w1473 w1529] -> w1423
        tunnel: [w1430 w1443 w1475 w1531] -> w1422
        tunnel: w1421 -> [w1430 w1442 w1474 w1530]
        tunnel: ["" ("initial string") w1435 w1468 w1524] -> w1420
        tunnel: [FALSE w1434 w1467 w1523] -> w1419
        tunnel: w1418 -> [_ w1432 w1462 w1518]
        frame 0, Default {
        }
        frame 1 {
          n302 = Unbundle By Name(w1442) -> ("Stop.SP.MaxTime"=w1433:dbl, "Stop.SP.Max Time Cond"=w1439:dbl)
          n303 = Subtract(x=w1432, y=w1439) -> (x-y=w1436:dbl)
          n304 = Greater Or Equal?(x=w1436, y=w1433) -> (x >= y?=w1440:bool)
          n305 = call "Main - Seconds to Time (SubVI).vi"("Seconds"=w1433) -> ("Time string"=w1431:string)  [unwired: 9 in, 1 out]
          n306 = case shown="True" w1440 {
            tunnel: [w1449 w1455] -> w1444
            tunnel: w1438 -> [w1449 w1454]
            tunnel: [w1447 w1460] -> w1443
            tunnel: w1442 -> [w1447 w1457]
            tunnel: [RunTest_-_State."Check Log" RunTest_-_State."Log"] -> w1441
            tunnel: "Stop Condition meet where Time >= %s" -> [_ w1453]
            tunnel: w1431 -> [_ w1452]
            tunnel: ["" w1451] -> w1435
            tunnel: [FALSE TRUE] -> w1434
            frame False {
            }
            frame True {
              n307 = Bundle By Name(cluster=w1457, "Running?"=FALSE) -> (w1460:T2)
              n308 = Format Into String(format string=w1453, initial string="", error in=w1454, w1452) -> (resulting string=w1451:string, error out=w1455:errorcluster)
            }
          }
        }
        frame 2 {
          n309 = Unbundle By Name(w1474) -> ("Stop.SP.Time"=w1461:dbl, "Stop.SP.Time Cond"=w1465:dbl, "Stop.SP.MaxTime"=w1466:dbl, "Stop.SP.Max Time Cond"=w1471:dbl)
          n310 = Subtract(x=w1462, y=w1465) -> (x-y=w1464:dbl)
          n311 = Subtract(x=w1462, y=w1471) -> (x-y=w1469:dbl)
          n312 = Greater Or Equal?(x=w1464, y=w1461) -> (x >= y?=w1463:bool)
          n313 = Greater Or Equal?(x=w1469, y=w1466) -> (x >= y?=w1472:bool)
          n314 = case shown="True" w1463 {
            tunnel: [w1479 w1490] -> w1476
            tunnel: [w1481 w1493] -> w1475
            tunnel: w1474 -> [w1481 w1492]
            tunnel: [RunTest_-_State."Check Log" w1486] -> w1473
            tunnel: w1472 -> [_ _]
            tunnel: w1470 -> [w1479 w1489]
            tunnel: ["" w1488] -> w1468
            tunnel: [FALSE w1487] -> w1467
            tunnel: w1466 -> [_ _]
            tunnel: w1462 -> [_ w1491]
            tunnel: w1461 -> [_ w1483]
            frame False {
            }
            frame True {
              n315 = Unbundle By Name(w1492) -> ("Sensor Data"=w1497:sgl[], "Stop.SP.Stress"=w1495:dbl)
              n316 = call "Main - Seconds to Time (SubVI).vi"("Seconds"=w1483) -> ("Time string"=w1482:string)  [unwired: 9 in, 1 out]
              n317 = Index Array(array=w1497, index=1) -> (element=w1484:sgl)
              n318 = Less Or Equal?(x=w1484, y=w1495) -> (x <= y?=w1494:bool)
              n319 = case shown="True" w1494 {
                tunnel: [w1503 w1509] -> w1493
                tunnel: w1492 -> [w1504 w1508]
                tunnel: w1491 -> [w1502 _]
                tunnel: [w1501 w1513] -> w1490
                tunnel: w1489 -> [w1501 w1514]
                tunnel: ["" w1512] -> w1488
                tunnel: [FALSE TRUE] -> w1487
                tunnel: [RunTest_-_State."Check Log" RunTest_-_State."Log"] -> w1486
                tunnel: "Stop Condition meet where Stress Changes <= %f after %s" -> [_ w1507]
                tunnel: w1484 -> [_ w1506]
                tunnel: w1482 -> [_ w1505]
                frame False {
                  n320 = Bundle By Name(cluster=w1504, "Stop.SP.Time Cond"=w1502) -> (w1503:T2)
                }
                frame True {
                  n321 = Bundle By Name(cluster=w1508, "Running?"=FALSE) -> (w1509:T2)
                  n322 = Format Into String(format string=w1507, initial string="", error in=w1514, w1506, w1505) -> (resulting string=w1512:string, error out=w1513:errorcluster)
                }
              }
            }
          }
        }
        frame 3 {
          n323 = Unbundle By Name(w1530) -> ("Stop.SP.Time"=w1517:dbl, "Stop.SP.Time Cond"=w1521:dbl, "Stop.SP.MaxTime"=w1522:dbl, "Stop.SP.Max Time Cond"=w1527:dbl)
          n324 = Subtract(x=w1518, y=w1521) -> (x-y=w1520:dbl)
          n325 = Subtract(x=w1518, y=w1527) -> (x-y=w1525:dbl)
          n326 = Greater Or Equal?(x=w1520, y=w1517) -> (x >= y?=w1519:bool)
          n327 = Greater Or Equal?(x=w1525, y=w1522) -> (x >= y?=w1528:bool)
          n328 = case shown="True" w1519 {
            tunnel: [w1543 w1568] -> w1532
            tunnel: [w1542 w1571] -> w1531
            tunnel: w1530 -> [w1541 w1570]
            tunnel: [w1540 w1564] -> w1529
            tunnel: w1528 -> [w1539 _]
            tunnel: w1526 -> [w1538 w1567]
            tunnel: [w1536 w1566] -> w1524
            tunnel: [w1535 w1565] -> w1523
            tunnel: w1522 -> [w1534 _]
            tunnel: w1518 -> [_ w1569]
            tunnel: w1517 -> [_ w1561]
            frame False {
              n329 = call "Main - Seconds to Time (SubVI).vi"("Seconds"=w1534) -> ("Time string"=w1533:string)  [unwired: 9 in, 1 out]
              n330 = case shown="True" w1539 {
                tunnel: [w1548 w1554] -> w1543
                tunnel: w1538 -> [w1548 w1553]
                tunnel: [w1546 w1559] -> w1542
                tunnel: w1541 -> [w1546 w1556]
                tunnel: [RunTest_-_State."Check Log" RunTest_-_State."Log"] -> w1540
                tunnel: "Stop Condition meet where Time >= %s" -> [_ w1552]
                tunnel: w1533 -> [_ w1551]
                tunnel: ["" w1550] -> w1536
                tunnel: [FALSE FALSE] -> w1535
                frame False {
                }
                frame True {
                  n331 = Bundle By Name(cluster=w1556, "Running?"=FALSE) -> (w1559:T2)
                  n332 = Format Into String(format string=w1552, initial string="", error in=w1553, w1551) -> (resulting string=w1550:string, error out=w1554:errorcluster)
                }
              }
            }
            frame True {
              n333 = Unbundle By Name(w1570) -> ("Sensor Data"=w1575:sgl[], "Stop.SP.Stress"=w1573:dbl)
              n334 = call "Main - Seconds to Time (SubVI).vi"("Seconds"=w1561) -> ("Time string"=w1560:string)  [unwired: 9 in, 1 out]
              n335 = Index Array(array=w1575, index=1) -> (element=w1562:sgl)
              n336 = Less Or Equal?(x=w1562, y=w1573) -> (x <= y?=w1572:bool)
              n337 = case shown="True" w1572 {
                tunnel: [w1581 w1587] -> w1571
                tunnel: w1570 -> [w1582 w1586]
                tunnel: w1569 -> [w1580 _]
                tunnel: [w1579 w1591] -> w1568
                tunnel: w1567 -> [w1579 w1592]
                tunnel: ["" w1590] -> w1566
                tunnel: [FALSE TRUE] -> w1565
                tunnel: [RunTest_-_State."Check Log" RunTest_-_State."Log"] -> w1564
                tunnel: "Stop Condition meet where Stress Changes <= %f after %s" -> [_ w1585]
                tunnel: w1562 -> [_ w1584]
                tunnel: w1560 -> [_ w1583]
                frame False {
                  n338 = Bundle By Name(cluster=w1582, "Stop.SP.Time Cond"=w1580) -> (w1581:T2)
                }
                frame True {
                  n339 = Bundle By Name(cluster=w1586, "Running?"=FALSE) -> (w1587:T2)
                  n340 = Format Into String(format string=w1585, initial string="", error in=w1592, w1584, w1583) -> (resulting string=w1590:string, error out=w1591:errorcluster)
                }
              }
            }
          }
        }
      }
    }
  }
  "Enum" <- w1
  n341 = Unbundle By Name(w2) -> ("fileid"=w9:string, "Test Plan"=w12:string[], "PlanRow"=w13:i32)
  n342 = Index Array(array=w12, index=w13) -> (element=w14:string)
  n343 = case shown="True" w11 {
    tunnel: w7 -> [w1595 w1602]
    tunnel: [w1595 w1601] -> w8
    tunnel: w9 -> [_ w1600]
    tunnel: w10 -> [_ w1596]
    tunnel: w14 -> [_ w1599]
    frame False {
    }
    frame True {
      n344 = Concatenate Strings(w1599, " | " ("string"), w1596) -> (w1597:string)
      n345 = call "Main - Event Log (eFGV).vi"("Action"=eFGV_States."Write", "error in"=w1602, "Fileid"=w1600, "Data In"=w1597) -> ("error out"=w1601:errorcluster)  [unwired: 4 in, 3 out]
    }
  }
  "error out" <- w8
  n346 = case shown="Default" w1 {
    tunnel: [w1604 w1606] -> w3
    tunnel: w2 -> [w1604 w1605]
    frame Default {
    }
    frame "Log" {
      n347 = Bundle By Name(cluster=w1605, "Last Log"=TRUE) -> (w1606:T2)
    }
  }
  "Cluster out" <- w3
